vi "rio 9030 jiwon.vi"() -> ()   [LabVIEW 2015]
uses:
  <vilib>/FPGAPlugInAG/cRIO-9030/niLvFpga_Open_cRIO-9030.vi
  <vilib>/rvi/interface/common/dynamic/niFpgaDynamicAddResources.vi
  <vilib>/FPGAPlugInAG/Dynamic/niLvFpga_Abort_Dynamic.vi
  <vilib>/FPGAPlugInAG/Dynamic/niLvFpga_Run_Dynamic.vi
  rio_Global.vi
  <vilib>/Utility/error.llb/Error Cluster From Error Code.vi
  <vilib>/rvi/errors/niLvFpgaAdjustHostInterfaceError.vi
  <vilib>/Analysis/Matrix/Numeric/Conversions/Array To Matrix - RA2.vi
  <vilib>/Analysis/Matrix/Numeric/Multiply/Multiply - RM,RM.vi
  <vilib>/Analysis/Matrix/Numeric/Add/Add - RM,RM.vi
  <vilib>/Analysis/baseanly.llb/Real Inverse Matrix.vi
  <vilib>/Analysis/Matrix/Numeric/Subtract/Subtract - RM,RM.vi
  <vilib>/Analysis/Matrix/Numeric/Conversions/Array To Matrix - RA.vi
  <vilib>/Analysis/Matrix/Numeric/Multiply/Multiply - R,RM.vi
  <vilib>/Analysis/Matrix/Numeric/Conversions/Matrix To Array - RM.vi
  <vilib>/rvi/interface/nirviOpenFPGA/nirviOpenFPGA.xnode
  FPGA Bitfiles/autonomous_FPGATarget4_fpga1_rudp+OsNkSQ.lvbitx
  samsung/fpga 1.vi
  <vilib>/rvi/interface/nirviMethod/nirviMethod.xnode
  <vilib>/rvi/interface/nirviReadWriteControl/nirviReadWriteControl.xnode
  <vilib>/FPGAPlugInAG/Dynamic/niLvFpga_ReadFifo_Dynamic.vi
  <vilib>/rvi/errors/niLvFpgaMergeErrorWithErrorCode.vi
  <vilib>/Analysis/Matrix/NI_Matrix.lvlib
  <vilib>/Analysis/NI_AALBase.lvlib
  <vilib>/rvi/interface/Simulation/niFpgaSimulationCallBeginRW.vi
  NiFpgaLv.dll
  <vilib>/addons/control/pid/NI_PID_pid.lvlib
  <vilib>/ptbypt/NI_PtbyPt.lvlib
  <vilib>/addons/control/pid/pid.llb/PID (DBL).vi
panel:
  in  "s":bool
  in  "Radio Buttons":enum32{"-480", "0", "480"}(radio)
  in  "Ref_str_ang":dbl
  out "error":dbl
  in  "STEERING PID_gain_Avante":dbl[](array[numeric])=[0.02, 6.5, 0.003]
  in  "STEERING PID_gain_Santafe":dbl[](array[numeric])=[0.02, 6.5, 0.003]
  out "map name":T1(ring)=enum."KAIST"
  out "Waveform Chart 3":dbl(graph)
  in  "lpf gain 2":dbl=0.8 format="%#_13g"
  out "con_dt":dbl
  in  "lpf gain":dbl=0.8 format="%#_13g"
  out "Waveform Chart 2":dbl(graph)
  in  "Dial":dbl(knob) min=-360.0 max=360.0 step=5.0 scale=-360.0..360.0
  out "FPGA":refnum<k20>
  out "C_yaw_rate":dbl
  in  "speed control":bool
  out "C_MCP":dbl
  out "C_APV":dbl
  out "Ref_VS":dbl
  out "XY Graph":cluster{"Y":dbl[], "Y":dbl[]}[](graph)=[{"Y"=[1.82421875, 1.8301353427767753, 1.835194070339203, 1.8394013252854347, 1.8427635002136231, 1.84528698772192, 1.8469781804084777, 1.8478434708714486, 1.8478892517089844, 1.8471219155192375, 1.84554785490036, 1.8431734624505043, 1.8400051307678222, 1.8360492524504661, 1.8313122200965881, 1.8258004263043404, 1.819520263671875, 1.8124781247973443, 1.8046804022789003, 1.796133488714695, 1.7868437767028809, 1.77681765884161, 1.7660615277290344, 1.7545817759633064, 1.742384796142578, 1.7294769808650017, 1.7158647227287291, 1.701554414331913, 1.686552448272705, 1.6708652171492577, 1.654499113559723, 1.637460530102253, 1.619755859375, 1.6013914939761162, 1.5823738265037537, 1.5627092495560646, 1.5424041557312012, 1.5214649376273155, 1.4998979878425598, 1.4777096989750862, 1.4549064636230469, 1.431494674384594, 1.4074807238578795, 1.3828710046410562, 1.3576719093322753, 1.3318898305296898, 1.3055311608314515, 1.2786022928357124, 1.251109619140625, 1.2230595323443412], "Y"=[0.0, 0.5, 1.0, 1.5, 2.0, 2.5, 3.0, 3.5, 4.0, 4.5, 5.0, 5.5, 6.0, 6.5, 7.0, 7.5, 8.0, 8.5, 9.0, 9.5, 10.0, 10.5, 11.0, 11.5, 12.0, 12.5, 13.0, 13.5, 14.0, 14.5, 15.0, 15.5, 16.0, 16.5, 17.0, 17.5, 18.0, 18.5, 19.0, 19.5, 20.0, 20.5, 21.0, 21.5, 22.0, 22.5, 23.0, 23.5, 24.0, 24.5]}, {"Y"=[-1.22265625, -1.2167396572232247, -1.211680929660797, -1.2074736747145653, -1.2041114997863769, -1.20158801227808, -1.1998968195915223, -1.1990315291285514, -1.1989857482910156, -1.1997530844807625, -1.20132714509964, -1.2037015375494957, -1.2068698692321778, -1.2108257475495339, -1.2155627799034119, -1.2210745736956596, -1.227354736328125, -1.2343968752026557, -1.2421945977210997, -1.250741511285305, -1.2600312232971191, -1.27005734115839, -1.2808134722709656, -1.2922932240366936, -1.304490203857422, -1.3173980191349983, -1.3310102772712709, -1.345320585668087, -1.360322551727295, -1.3760097828507423, -1.392375886440277, -1.409414469897747, -1.427119140625, -1.4454835060238838, -1.4645011734962463, -1.4841657504439354, -1.5044708442687988, -1.5254100623726845, -1.5469770121574402, -1.5691653010249138, -1.5919685363769531, -1.615380325615406, -1.6393942761421205, -1.6640039953589438, -1.6892030906677247, -1.7149851694703102, -1.7413438391685485, -1.7682727071642876, -1.795765380859375, -1.8238154676556588, -1.8524165749549866, -1.8815623101592065, -1.911246280670166, -1.9414620938897134, -1.972203357219696, -2.003463678061962, -2.0352366638183597, -2.0675159218907355, -2.1002950596809384, -2.1335676845908162, -2.167327404022217, -2.2015678253769875, -2.2362825560569766, -2.2714652034640315, -2.307109375, -2.3432086780667305, -2.3797567200660703, -2.4167471083998677, -2.4541734504699706, -2.4920293536782263, -2.530308425426483, -2.5690042731165885, -2.6081105041503907, -2.647620725929737, -2.687528545856476, -2.7278275713324547, -2.7685114097595216, -2.809573668539524, -2.8510079550743104, -2.892807876765728, -2.934967041015625, -2.977479055225849, -3.020337526798248, -3.0635360631346704, -3.107068271636963, -3.150927759706974, -3.1951081347465515, -3.2396030041575434, -3.284405975341797, -3.3295106557011604, -3.3749106526374817, -3.4205995735526087, -3.466571025848389, -3.51281861692667, -3.5593359541893004], "Y"=[0.0, 0.5, 1.0, 1.5, 2.0, 2.5, 3.0, 3.5, 4.0, 4.5, 5.0, 5.5, 6.0, 6.5, 7.0, 7.5, 8.0, 8.5, 9.0, 9.5, 10.0, 10.5, 11.0, 11.5, 12.0, 12.5, 13.0, 13.5, 14.0, 14.5, 15.0, 15.5, 16.0, 16.5, 17.0, 17.5, 18.0, 18.5, 19.0, 19.5, 20.0, 20.5, 21.0, 21.5, 22.0, 22.5, 23.0, 23.5, 24.0, 24.5, 25.0, 25.5, 26.0, 26.5, 27.0, 27.5, 28.0, 28.5, 29.0, 29.5, 30.0, 30.5, 31.0, 31.5, 32.0, 32.5, 33.0, 33.5, 34.0, 34.5, 35.0, 35.5, 36.0, 36.5, 37.0, 37.5, 38.0, 38.5, 39.0, 39.5, 40.0, 40.5, 41.0, 41.5, 42.0, 42.5, 43.0, 43.5, 44.0, 44.5, 45.0, 45.5, 46.0, 46.5, 47.0]}, {"Y"=[-0.94, 0.94, 0.94, -0.94, -0.94], "Y"=[-3.2, -3.2, 1.5, 1.5, -3.2]}, {"Y"=[1.984375, 1.978057861328125, 1.9718017578125, 1.965606689453125, 1.95947265625], "Y"=[0.0, 0.5, 1.0, 1.5, 2.0]}, {"Y"=[-5.28125, -5.267578125, -5.25390625, -5.240234375, -5.2265625], "Y"=[0.0, 0.5, 1.0, 1.5, 2.0]}]
  out "x_view":dbl[](array[numeric])=[0.0, 0.5, 1.0, 1.5, 2.0, 2.5, 3.0, 3.5, 4.0, 4.5, 5.0, 5.5, 6.0, 6.5, 7.0, 7.5, 8.0, 8.5, 9.0, 9.5, 10.0, 10.5, 11.0, 11.5, 12.0, 12.5, 13.0, 13.5, 14.0, 14.5, 15.0, 15.5, 16.0, 16.5, 17.0, 17.5, 18.0, 18.5, 19.0, 19.5, 20.0, 20.5, 21.0, 21.5, 22.0, 22.5, 23.0, 23.5, 24.0, 24.5, 25.0, 25.5, 26.0, 26.5, 27.0, 27.5, 28.0, 28.5, 29.0, 29.5, 30.0, 30.5, 31.0, 31.5, 32.0, 32.5, 33.0, 33.5, 34.0, 34.5, 35.0, 35.5, 36.0, 36.5, 37.0, 37.5, 38.0, 38.5, 39.0, 39.5, 40.0, 40.5, 41.0, 41.5, 42.0, 42.5, 43.0, 43.5, 44.0, 44.5, 45.0, 45.5, 46.0, 46.5, 47.0, 47.5, 48.0, 48.5, 49.0, 49.5, 50.0, 50.5, 51.0, 51.5, 52.0, 52.5, 53.0, 53.5, 54.0, 54.5, 55.0, 55.5, 56.0, 56.5, 57.0, 57.5, 58.0, 58.5, 59.0, 59.5, 60.0, 60.5, 61.0, 61.5, 62.0, 62.5, 63.0, 63.5, 64.0, 64.5, 65.0, 65.5, 66.0, 66.5, 67.0, 67.5, 68.0, 68.5, 69.0, 69.5, 70.0, 70.5, 71.0, 71.5, 72.0, 72.5, 73.0, 73.5, 74.0, 74.5, 75.0, 75.5, 76.0, 76.5, 77.0, 77.5, 78.0, 78.5, 79.0, 79.5, 80.0, 80.5, 81.0, 81.5, 82.0, 82.5, 83.0, 83.5, 84.0, 84.5, 85.0, 85.5, 86.0, 86.5, 87.0, 87.5, 88.0, 88.5, 89.0, 89.5, 90.0, 90.5, 91.0, 91.5, 92.0, 92.5, 93.0, 93.5, 94.0, 94.5, 95.0, 95.5, 96.0, 96.5, 97.0, 97.5, 98.0, 98.5, 99.0, 99.5, 100.0, 100.5, 101.0, 101.5, 102.0, 102.5, 103.0, 103.5, 104.0, 104.5, 105.0, 105.5, 106.0, 106.5, 107.0, 107.5, 108.0, 108.5, 109.0, 109.5, 110.0, 110.5, 111.0, 111.5, 112.0, 112.5, 113.0, 113.5, 114.0, 114.5, 115.0, 115.5, 116.0, 116.5, 117.0, 117.5, 118.0, 118.5, 119.0, 119.5, 120.0, 120.5, 121.0, 121.5, 122.0, 122.5, 123.0, 123.5, 124.0, 124.5, 125.0, 125.5, 126.0, 126.5, 127.0, 127.5, 128.0]
  in  "Manual Steering torque":dbl(slide) min=-0.9 max=0.9 step=0.01 scale=-0.9..0.9
  out "T init":i32
  out "T out":i32
  out "PWM GAS":dbl=1000.0 min=1000.0 max=2000.0 step=1.0
  out "Mobileye_time 50":u32
  out "H_GPS":dbl
  out "vgain":dbl=1.0
  out "vcount":u64=1
  out "hbias":dbl
  out "hcount":u64=1
  out "get heading":bool
  out "get position":bool
  out "heading error":dbl
  out "h_gps":dbl
  out "rt":dbl
  out "pos error":dbl
  out "POS init":bool
  out "Heading":dbl
  out "pos":dbl[](array[numeric])
  in  "GPS init":bool=TRUE
  out "pos_gps":dbl[](array[numeric]) format="%#_19f"
  out "dt":dbl
  out "Pos_time 10":i32
  out "ecef ref":dbl[](array[numeric])
  in  "Velocity input":bool
  in  "Manual Speed":dbl=1.0
  in  "Steer input":bool=TRUE
  out "Run":bool
  out "Auto":bool
  out "E - STOP":bool
  out "Con_time 10":i32
  out "VS_CAN":dbl
  out "CAN_time 10":u32
  out "gps1":refnum<visa-resource-name>
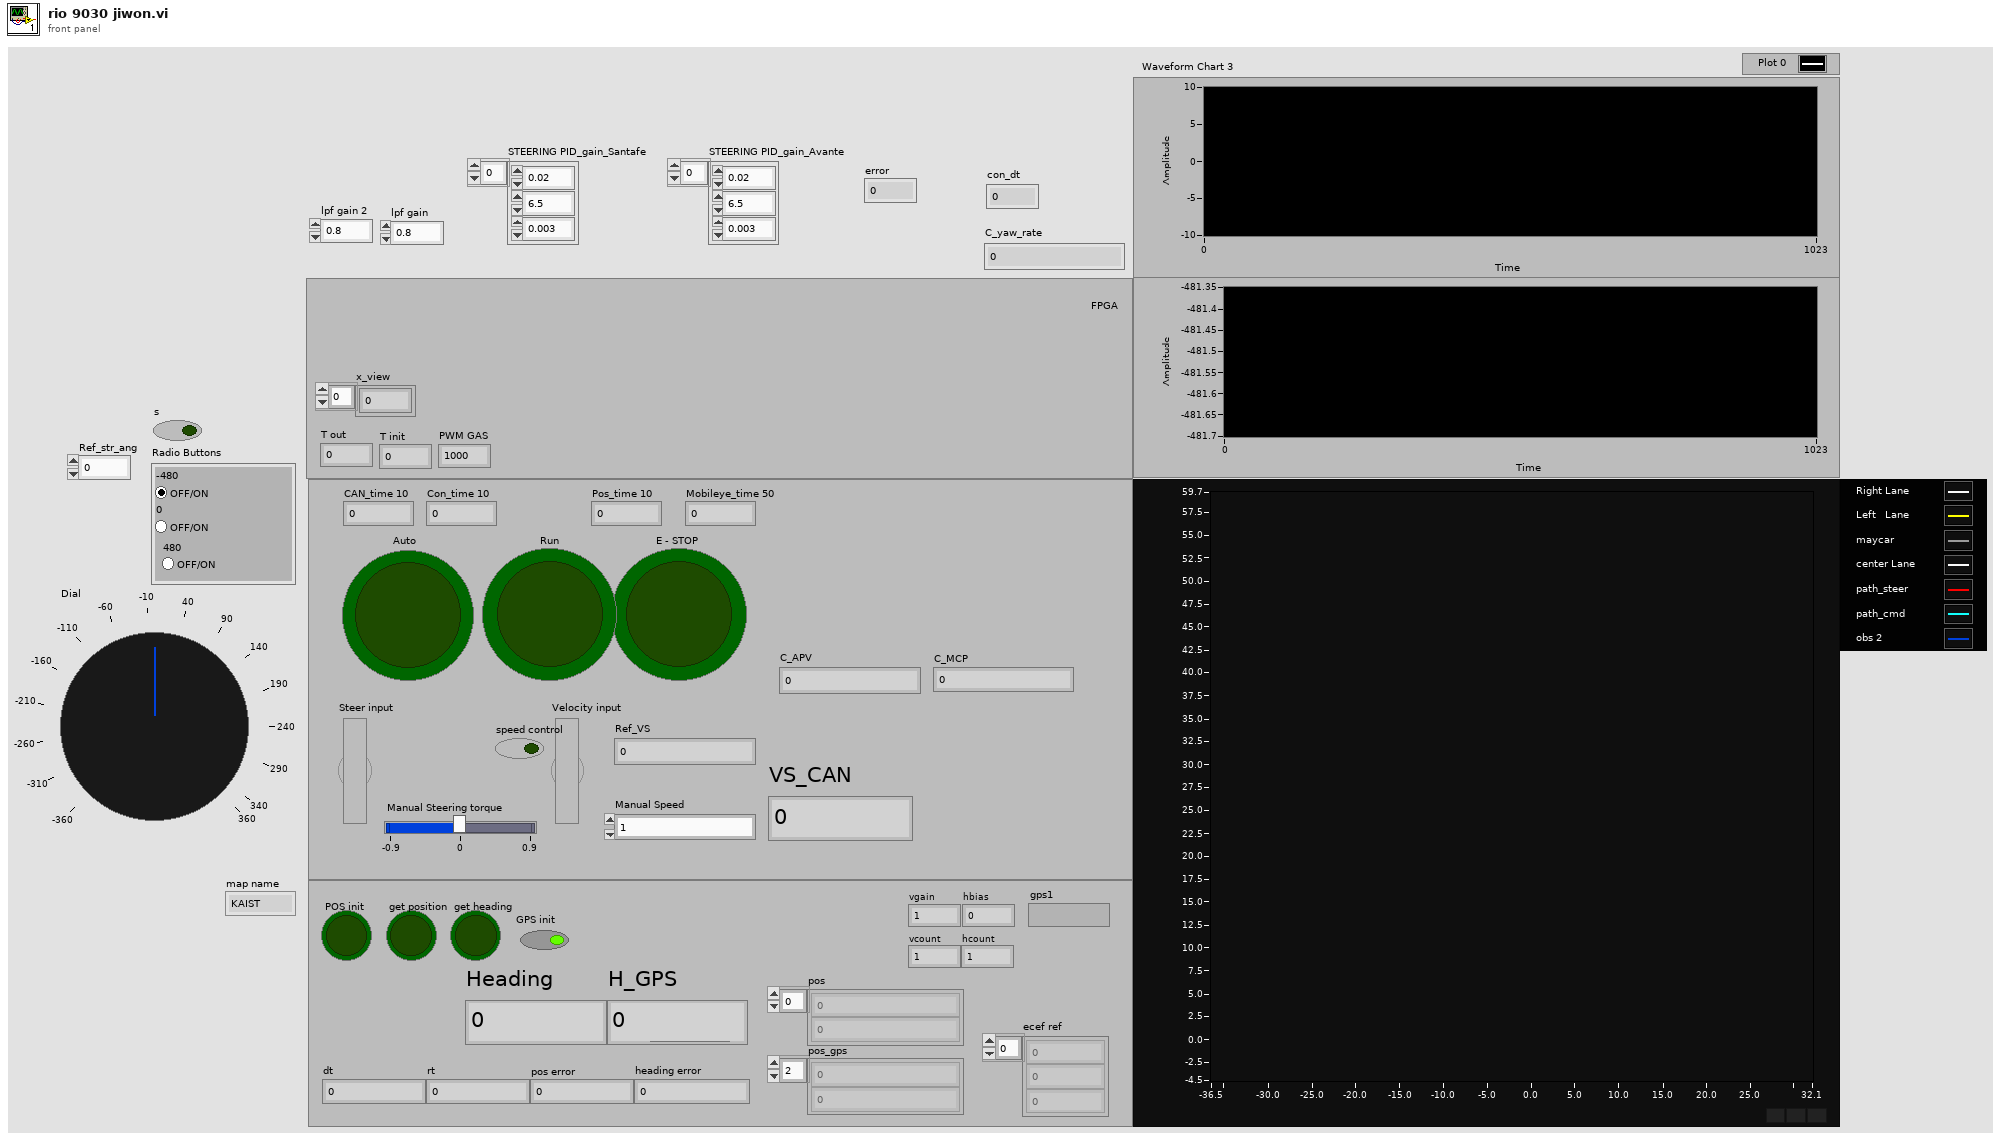
[diagram p1: front panel]
types:
  T1 = enum32{"Namyang", "Hyundai", "KAIST", "Ajou", "Munji", "Airforce", "Car", "KATRI", "Samsung", "Coex", "Gwangnaru", "Inje", "sinjin"}
  T2 = cluster{"proportional gain (Kc)":dbl, "integral time (Ti, min)":dbl, "derivative time (Td, min)":dbl}
  T3 = cluster{"connection ID":refnum<k16>, "net address":u32, "port":u16}
  T4 = cluster{"hash":i64, "sys time":i64, "ref_vel":dbl, "ref_steer":dbl, "alert":u8}
  T5 = cluster{"hash":i64, "sys time":i64, "ref_vel":dbl, "ref_steer":dbl}
  T6 = cluster{"hash":i64, "sys time":i64, "Auto":bool, "Run":bool, "Solenoid":bool, "T lim":bool, "brk_enc":u8, "B PWM":u16, "T PWM":u16, "ref_vel":dbl, "ref_bkr_enc":dbl, "ref_apv":dbl, "ref_steer":dbl, "net address":u32}
  T7 = cluster{"identifier":u32, "timestamp":timestamp, "payload":u8[]}
  T8 = cluster{"timestamp high":u32, "timestamp low":u32, "identifier":u32, "type":enum8{"Data Frame", "Remote Frame", "(reserved)", "(reserved) ", "(reserved)  ", "(reserved)   ", "Bus Error", "Transceiver Fault"}, "info A":u8, "info B":u8, "data length":u8, "data":u8[]}
  T9 = cluster{"hash":i64, "sys time":i64, "size":i32, "data":u8[]}
  T10 = cluster{"hash":i64, "sys time":i64, "time":dbl, "yaw_rate":dbl, "mdps torque":dbl, "mdps str_ang":dbl, "VS_CAN":dbl, "lat_accel":dbl, "mcp":dbl, "accel pedal value":dbl, "tps":dbl, "odometer":dbl, "battery voltage":dbl, "WHL_SPD_RR":dbl, "WHL_SPD_RL":dbl, "WHL_SPD_FR":dbl, "WHL_SPD_FL":dbl}
  T11 = typedef "NI_Matrix.lvlib/RealMatrix.ctl" = dbl[][]
  T12 = cluster{"hash":i64, "sys time":i64, "dt":dbl, "x":dbl, "y":dbl, "speed":dbl, "heading":dbl, "yaw_rate":dbl}
  T13 = cluster{"Real 2D Array[0]":dbl, "Real 2D Array[1]":dbl, "Real 2D Array[2]":dbl, "Real 2D Array[3]":dbl, "Real 2D Array[4]":dbl}
  T14 = cluster{"hash":i64, "sys time":i64, "time":dbl, "x":dbl, "y":dbl, "h":dbl, "numSV":i32, "postype":i32, "lag":i32, "hordev":dbl, "lat":dbl, "lon":dbl, "hgt":dbl, "map_idx":i32}
  T15 = cluster{"output[0]":dbl, "output[1]":dbl, "output[2]":dbl, "output[3]":dbl, "output[4]":dbl, "output[5]":dbl, "output[6]":dbl, "output[7]":dbl, "output[8]":dbl, "output[9]":dbl, "output[10]":dbl, "output[11]":dbl, "output[12]":dbl, "output[13]":dbl, "output[14]":dbl}
  T16 = cluster{"hash":i64, "sys time":i64, "time":dbl, "speed":dbl, "heading":dbl, "lat":dbl, "lon":dbl}
  T17 = cluster{"output[0]":dbl, "output[1]":dbl, "output[2]":dbl, "output[3]":dbl, "output[4]":dbl, "output[5]":dbl, "output[6]":dbl}
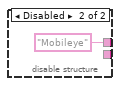
[diagram p2: hidden frame]
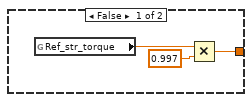
[diagram p3: hidden frame]
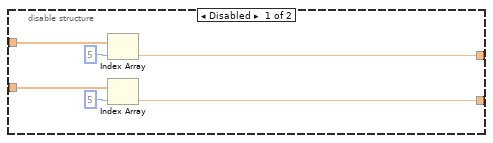
[diagram p4: hidden frame]
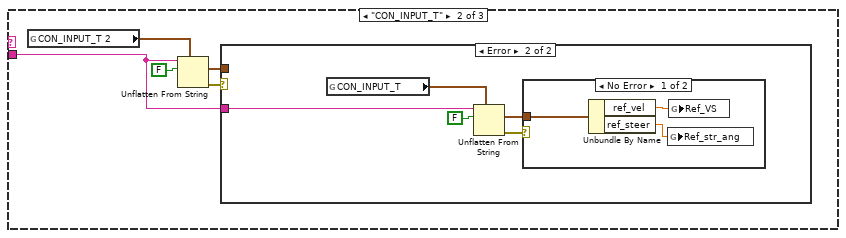
[diagram p6: hidden frame]
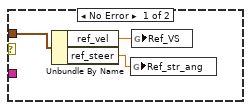
[diagram p7: hidden frame]
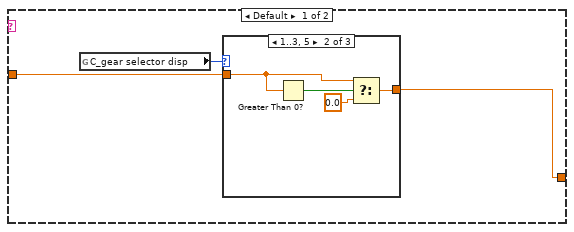
[diagram p10: hidden frame]
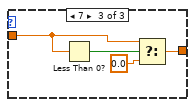
[diagram p12: hidden frame]
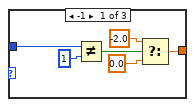
[diagram p13: hidden frame]
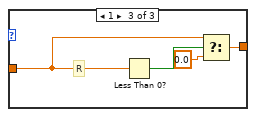
[diagram p16: hidden frame]
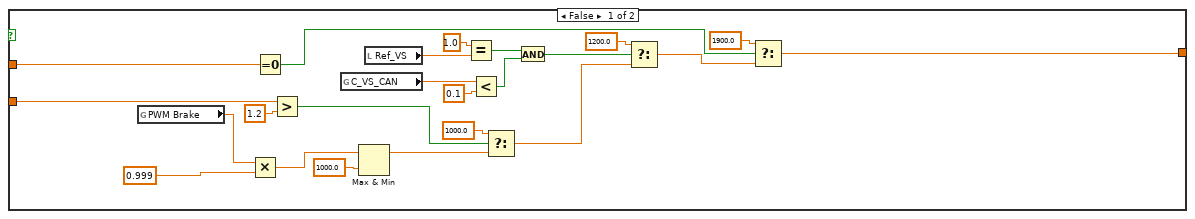
[diagram p17: hidden frame]
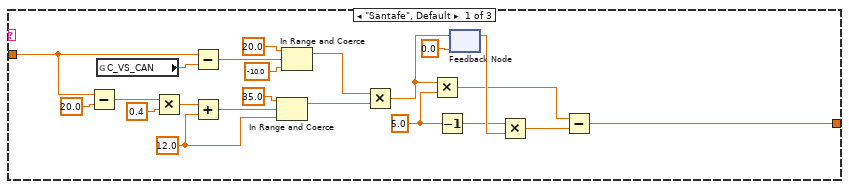
[diagram p19: hidden frame]
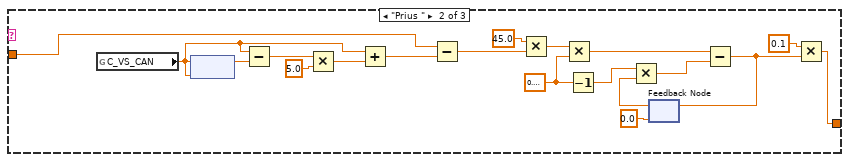
[diagram p20: hidden frame]
diagram:
  n1 = flat-sequence {
    frame #0 {
      n2 = local write "Manual Steering torque"(0.0 ("Ref_vel_planner")) -> ()
      n3 = local write "Velocity input"(FALSE ("GPS init")) -> ()
      n4 = local write "Steer input"(FALSE ("Steer input")) -> ()
      n5 = local write "Manual Speed"(20.0 ("manual Speed")) -> ()
      n6 = global write "rio_Global.vi" "lane width"(3.5 ("lane width")) -> ()
    }
    frame #1 {
      n7 = while {
        stop <- FALSE stop-if-true
        n8 = flat-sequence {
          tunnel: [w127] -> w7
          tunnel: w7 -> [w180]
          frame #0 {
            n9 = Wait Until Next ms Multiple(millisecond multiple=u32 10) -> (millisecond timer value=w12:u32)
            n10 = feedback #1(w12) -> (w11:u32)
            n11 = feedback-in #1(w12) -> ()
            n12 = Subtract(x=w12, y=w11) -> (x-y=w10:u32)
            n13 = To Long Integer(number=w10) -> (32bit integer=→"Con_time 10":i32)
          }
          frame #1 {
            n14 = disable-structure shown="Enabled" {
              disable-tunnel: [w17 "Mobileye" ("ID")] -> w15
              disable-tunnel: [w16 _] -> w14
              frame Enabled {
                n15 = global read "rio_Global.vi" "LCM PC"() -> (w18:T3)
                n16 = call "LCM_read.vi"("LCM"=w18) -> ("data"=w16:string, "ID"=w17:string)  [unwired: 7 in, 2 out]
              }
              frame Disabled {
              }
            }
            n17 = case shown="\"Mobileye\"" w15 {
              tunnel: w14 -> [_ w111 _]
              frame "Mobileye" {
                n18 = flat-sequence {
                  frame #0 {
                    w26 = 2 ("index")
                    w29 = 2 ("index")
                    n19 = global read "rio_Global.vi" "M_lane_right"() -> (w21:dbl[])
                    n20 = global read "rio_Global.vi" "M_lane_left"() -> (w22:dbl[])
                    n21 = Index Array(array=w22, index=w29) -> (element=w28:dbl)
                    n22 = Index Array(array=w21, index=w26) -> (element=w27:dbl)
                    n23 = Greater Or Equal?(x=w28, y=w29) -> (x >= y?=w23:bool)
                    n24 = Greater Or Equal?(x=w27, y=w26) -> (x >= y?=w24:bool)
                    n25 = Or(x=w23, y=w24) -> (x .or. y?=w25:bool)
                    n26 = case shown="True" w25 {
                      tunnel: w24 -> [_ w57]
                      tunnel: [w30 w46] -> w20
                      tunnel: w23 -> [_ w60]
                      tunnel: w22 -> [_ w51]
                      tunnel: w21 -> [_ w50]
                      frame False {
                        n27 = global read "rio_Global.vi" "Ref_str_torque"() -> (w31:dbl)
                        n28 = Multiply(x=w31, y=0.997) -> (x*y=w30:dbl)
                      }
                      frame True {
                        n29 = disable-structure shown="Enabled" {
                          disable-tunnel: [w65 w68] -> w56
                          disable-tunnel: [w64 w90] -> w54
                          disable-tunnel: w51 -> [w63 w99]
                          disable-tunnel: w50 -> [w62 w69]
                          frame Disabled {
                            n30 = Index Array(array=w63, index=5) -> (element=w64:dbl)
                            n31 = Index Array(array=w62, index=5) -> (element=w65:dbl)
                          }
                          frame Enabled {
                            n32 = global read "rio_Global.vi" "C_VS_CAN"() -> (w98:dbl)
                            n33 = global read "rio_Global.vi" "C_VS_CAN"() -> (w74:dbl)
                            n34 = In Range and Coerce(upper limit=45.0, x=w98, lower limit=15.0) -> (coerced(x)=w87:dbl)  [unwired: 1 out]
                            n35 = In Range and Coerce(upper limit=45.0, x=w74, lower limit=15.0) -> (coerced(x)=w84:dbl)  [unwired: 1 out]
                            n36 = Index Array(array=w99, index #1=7 ("index"), index #2=6 ("index"), index #3=9 ("index"), index #4=5 ("index")) -> (element #1=w95:dbl, element #2=w88:dbl, element #3=w86:dbl, element #4=w91:dbl)
                            n37 = Index Array(array=w69, index #1=7 ("index"), index #2=6 ("index"), index #3=9 ("index"), index #4=5 ("index")) -> (element #1=w77:dbl, element #2=w83:dbl, element #3=w85:dbl, element #4=w81:dbl)
                            n38 = Square(x=w87) -> (x^2=w89:dbl)
                            n39 = Square(x=w84) -> (x^2=w82:dbl)
                            n40 = Multiply(x=w89, y=w88) -> (x*y=w93:dbl)
                            n41 = Multiply(x=w87, y=w86) -> (x*y=w92:dbl)
                            n42 = Multiply(x=w82, y=w83) -> (x*y=w79:dbl)
                            n43 = Multiply(x=w84, y=w85) -> (x*y=w80:dbl)
                            n44 = Compound Arithmetic op=MULTIPLY(w95, w89, w87) -> (w94:dbl)
                            n45 = Compound Arithmetic op=MULTIPLY(w77, w82, w84) -> (w78:dbl)
                            n46 = Compound Arithmetic op=ADD(w94, w93, w92, w91) -> (w90:dbl)
                            n47 = Compound Arithmetic op=ADD(w78, w79, w80, w81) -> (w68:dbl)
                          }
                        }
                        n48 = global read "rio_Global.vi" "C_VS_CAN"() -> (w49:dbl)
                        n49 = global read "rio_Global.vi" "lane width"() -> (w53:dbl)
                        n50 = Square(x=w49) -> (x^2=w48:dbl)
                        n51 = Add(x=w54, y=w53) -> (x+y=w52:dbl)
                        n52 = Subtract(x=w56, y=w53) -> (x-y=w58:dbl)
                        n53 = Divide(x=w48, y=-28800.0) -> (x/y=w45:dbl)
                        n54 = Select(t=w54, s=w60, f=w58) -> (s? t:f=w59:dbl)
                        n55 = Select(t=w56, s=w57, f=w52) -> (s? t:f=w55:dbl)
                        n56 = global read "rio_Global.vi" "C_Right light"() -> (w37:bool)
                        n57 = global read "rio_Global.vi" "C_Left light"() -> (w35:bool)
                        n58 = Negate(x=w59) -> (-x=w61:dbl)
                        n59 = Multiply(x=w45, y=4.499999999999998 ("invgain>1")) -> (x*y=w44:dbl)
                        n60 = Subtract(x=w61, y=w55) -> (x-y=w34:dbl)
                        n61 = Exclusive Or(1:w37, 2:w35) -> (0:w36:bool)
                        n62 = Exponential(1:w44) -> (0:w41:dbl)
                        n63 = case shown="True" w36 {
                          tunnel: w35 -> [_ w110]
                          tunnel: [w104 w105] -> w33
                          tunnel: w34 -> [w104 w107]
                          frame False {
                          }
                          frame True {
                            n64 = Select(t=1.0, s=w110, f=-1.0) -> (s? t:f=w106:dbl)
                            n65 = Add(x=w107, y=w106) -> (x+y=w105:dbl)
                          }
                        }
                        n66 = Multiply(x=w41, y=0.125) -> (x*y=w40:dbl)
                        n67 = Max & Min(x=w40, y=0.01) -> (max(x,y)=w39:dbl)  [unwired: 1 out]
                        n68 = Multiply(x=w33, y=w39) -> (x*y=w46:dbl)
                      }
                    }
                    n69 = global write "rio_Global.vi" "Ref_str_torque"(w20) -> ()
                  }
                }
              }
              frame "CON_INPUT_T" {
                n70 = global read "rio_Global.vi" "CON_INPUT_T 2"() -> (w113:T4)
                n71 = Unflatten From String(type=w113, binary string=w111, data includes array or string size? (T)=FALSE) -> (value=w112:T4, error out=w114:errorcluster)  [unwired: 2 in, 1 out]
                n72 = case shown="Error" w114 {
                  tunnel: w112 -> [w118 _]
                  tunnel: w111 -> [_ w119]
                  frame No Error {
                    n73 = Unbundle By Name(w118) -> ("ref_vel"=w117:dbl, "ref_steer"=w116:dbl)
                    n74 = global write "rio_Global.vi" "Ref_str_ang"(w116) -> ()
                    n75 = global write "rio_Global.vi" "Ref_VS"(w117) -> ()
                  }
                  frame Error {
                    n76 = global read "rio_Global.vi" "CON_INPUT_T"() -> (w121:T5)
                    n77 = Unflatten From String(type=w121, binary string=w119, data includes array or string size? (T)=FALSE) -> (value=w120:T5, error out=w122:errorcluster)  [unwired: 2 in, 1 out]
                    n78 = case shown="No Error" w122 {
                      tunnel: w120 -> [w126 _]
                      frame No Error {
                        n79 = Unbundle By Name(w126) -> ("ref_vel"=w125:dbl, "ref_steer"=w124:dbl)
                        n80 = global write "rio_Global.vi" "Ref_str_ang"(w124) -> ()
                        n81 = global write "rio_Global.vi" "Ref_VS"(w125) -> ()
                      }
                      frame Error {
                      }
                    }
                  }
                }
              }
              frame Default {
              }
            }
          }
          frame #2 {
            n82 = global read "rio_Global.vi" "C_VS_CAN"() -> (→"VS_CAN":dbl)
            n83 = global read "rio_Global.vi" "C_MCP"() -> (→"C_MCP":dbl)
            n84 = global read "rio_Global.vi" "Ref_VS"() -> (w128:dbl)
            n85 = global read "rio_Global.vi" "C_APV"() -> (→"C_APV":dbl)
            n86 = local read "Con_time 10"() -> (w134:i32)
            n87 = global read "rio_Global.vi" "Car_name"() -> (w129:string)
            n88 = Select(t=w128, s="Velocity input", f="Manual Speed") -> (s? t:f=w139:dbl)
            n89 = To Double Precision Float(number=w134) -> (double precision float=w135:dbl)
            n90 = case shown="\"Prius\"" w129 {
              tunnel: w139 -> [w143 w157]
              tunnel: [w142 w158] -> w127
              frame Default {
                n91 = global read "rio_Global.vi" "C_gear selector disp"() -> (w144:u8)
                n92 = case shown="1..3, 5" w144 {
                  tunnel: w143 -> [_ w147 w151]
                  tunnel: [_ w146 w150] -> w142
                  frame 0, Default {
                  }
                  frame 1..3, 5 {
                    n93 = Greater Than 0?(x=w147) -> (x > 0?=w148:bool)
                    n94 = Select(t=w147, s=w148, f=0.0) -> (s? t:f=w146:dbl)
                  }
                  frame 7 {
                    n95 = Less Than 0?(x=w151) -> (x < 0?=w152:bool)
                    n96 = Select(t=w151, s=w152, f=0.0) -> (s? t:f=w150:dbl)
                  }
                }
              }
              frame "Prius" {
                n97 = Sign(1:w157) -> (0:w156:dbl)
                n98 = global read "rio_Global.vi" "C_gear selector disp"() -> (w154:u8)
                n99 = To Long Integer(number=w156) -> (32bit integer=w155:i32)
                n100 = case shown="1" w155 {
                  tunnel: [w160 _ w166] -> w153
                  tunnel: w154 -> [w163 _ w169]
                  frame -1 {
                    n101 = Not Equal?(x=w163, y=u8 1) -> (x != y?=w162:bool)
                    n102 = Select(t=-2.0 ("element"), s=w162, f=0.0) -> (s? t:f=w160:dbl)
                  }
                  frame 0, Default {
                  }
                  frame 1 {
                    n103 = Not Equal?(x=w169, y=u8 3) -> (x != y?=w167:bool)
                    n104 = Select(t=2.0 ("element"), s=w167, f=0.0) -> (s? t:f=w166:dbl)
                  }
                }
                n105 = case shown="3" w154 {
                  tunnel: [_ w171 w176] -> w158
                  tunnel: w157 -> [_ w173 w177]
                  frame 0, Default {
                    # "P,N"
                  }
                  frame 3 {
                    # "D"
                    n106 = Greater Than 0?(x=w173) -> (x > 0?=w174:bool)
                    n107 = Select(t=w173, s=w174, f=0.0) -> (s? t:f=w171:dbl)
                  }
                  frame 1 {
                    # "R"
                    n108 = Less Than 0?(x=w177) -> (x < 0?=w178:bool)
                    n109 = Select(t=w177, s=w178, f=0.0) -> (s? t:f=w176:dbl)
                  }
                }
                n110 = global write "rio_Global.vi" "Shift control"(w153) -> ()
              }
            }
            "Ref_VS" <- w127
            n111 = Multiply(x=w135, y=0.001) -> (x*y=w133:dbl)
            n112 = Max & Min(x=w133, y=0.005) -> (max(x,y)=→"con_dt":dbl)  [unwired: 1 out]
          }
          frame #3 {
            n113 = flat-sequence {
              tunnel: [w192] -> w179
              tunnel: w180 -> [w193]
              frame #0 {
                n114 = global read "rio_Global.vi" "C_VS_CAN"() -> (w195:dbl)
                n115 = Subtract(x=w193, y=w195) -> (x-y=w194:dbl)
                n116 = Less?(x=w194, y=0.0 ("lower limit")) -> (x < y?=w196:bool)
                n117 = case shown="True" w196 {
                  tunnel: [w200 w225] -> w192
                  tunnel: w193 -> [w213 w236]
                  tunnel: w194 -> [w210 w228]
                  frame False {
                    n118 = global read "rio_Global.vi" "PWM Brake"() -> (w220:dbl)
                    n119 = Multiply(x=w220, y=0.999 ("brake relase gain")) -> (x*y=w219:dbl)
                    n120 = Equal To 0?(x=w213) -> (x = 0?=w212:bool)
                    n121 = Greater?(x=w210, y=1.2) -> (0:w217:bool)
                    n122 = global read "rio_Global.vi" "C_VS_CAN"() -> (w203:dbl)
                    n123 = Max & Min(x=w219, y=1000.0) -> (max(x,y)=w215:dbl)  [unwired: 1 out]
                    n124 = local read "Ref_VS"() -> (w208:dbl)
                    n125 = Equal?(x=1.0, y=w208) -> (x = y?=w206:bool)
                    n126 = Less?(x=w203, y=0.1 ("x")) -> (x < y?=w201:bool)
                    n127 = Select(t=1000.0, s=w217, f=w215) -> (s? t:f=w199:dbl)
                    n128 = And(x=w206, y=w201) -> (x .and. y?=w205:bool)
                    n129 = Select(t=1200.0, s=w205, f=w199) -> (s? t:f=w198:dbl)
                    n130 = Select(t=1900.0, s=w212, f=w198) -> (s? t:f=w200:dbl)
                  }
                  frame True {
                    w234 = 0.5 ("gain brake")
                    n131 = Absolute Value(x=w228) -> (abs(x)=w227:dbl)
                    n132 = Threshold 1D Array(2:w227, 3:dbl[] [0.1, 0.5, 1.0, 1.5, 2.0, 3.0, 4.0, 5.0, 6.0, 7.0, 8.0, 9.0, 10.0, 6.5, 7.0, 7.5, 8.0, 8.5, 9.0, 9.5, 10.0]) -> (0:w239:dbl)  [unwired: 1 in]
                    n133 = global read "rio_Global.vi" "PWM Brake"() -> (w232:dbl)
                    n134 = Interpolate 1D Array(1:w239, 2:dbl[] [1250.0, 1270.0, 1290.0, 1300.0, 1350.0, 1400.0, 1450.0, 1500.0, 1550.0, 1700.0, 1750.0, 1900.0, 1900.0]) -> (0:w235:dbl)
                    n135 = Decrement(x=w234) -> (x-1=w233:dbl)
                    n136 = Multiply(x=w235, y=w234) -> (x*y=w230:dbl)
                    n137 = Multiply(x=w233, y=w232) -> (x*y=w231:dbl)
                    n138 = Subtract(x=w230, y=w231) -> (x-y=w226:dbl)
                    n139 = disable-structure shown="Enabled" {
                      disable-tunnel: [w241 w242] -> w223
                      disable-tunnel: w226 -> [w241 w255]
                      disable-tunnel: w227 -> [_ w247]
                      frame Disabled {
                      }
                      frame Enabled {
                        n140 = Multiply(x=w247, y=120.0 ("brake p gain")) -> (x*y=w253:dbl)
                        n141 = local read "con_dt"() -> (w250:dbl)
                        n142 = Add(x=w255, y=w253) -> (x+y=w244:dbl)
                        n143 = Multiply(x=w250, y=4.0) -> (x*y=w249:dbl)
                        n144 = call <vilib>:"Derivative x(t) PtByPt.vi"("initialize"=FALSE, "dt"=w249, "initial condition"=0.0, "x"=w247) -> ("dx/dt"=w245:dbl)  [unwired: 1 out]
                        n145 = Multiply(x=30.0 ("bake d gain"), y=w245) -> (x*y=w243:dbl)
                        n146 = Add(x=w244, y=w243) -> (x+y=w242:dbl)
                      }
                    }
                    n147 = Equal To 0?(x=w236) -> (x = 0?=w237:bool)
                    n148 = In Range and Coerce(upper limit=1900.0, x=w223, lower limit=1000.0) -> (coerced(x)=w221:dbl)  [unwired: 1 out]
                    n149 = Select(t=1900.0, s=w237, f=w221) -> (s? t:f=w225:dbl)
                  }
                }
              }
            }
            n150 = global read "rio_Global.vi" "Car_name"() -> (w181:string)
            n151 = case shown="\"Avante\"" w181 {
              tunnel: [w277 w296 w322] -> w186
              tunnel: w180 -> [w276 w295 w321]
              frame "Santafe", Default {
                w260 = 5.0 ("gain accel")
                w268 = 12.0 ("y")
                n152 = Subtract(x=w276, y=20.0) -> (x-y=w272:dbl)
                n153 = global read "rio_Global.vi" "C_VS_CAN"() -> (w257:dbl)
                n154 = Multiply(x=w272, y=0.4) -> (x*y=w270:dbl)
                n155 = Subtract(x=w276, y=w257) -> (x-y=w256:dbl)
                n156 = Add(x=w270, y=w268) -> (x+y=w269:dbl)
                n157 = In Range and Coerce(upper limit=35.0, x=w269, lower limit=w268) -> (coerced(x)=w266:dbl)  [unwired: 1 out]
                n158 = In Range and Coerce(upper limit=20.0, x=w256, lower limit=-10.0) -> (coerced(x)=w265:dbl)  [unwired: 1 out]
                n159 = Multiply(x=w265, y=w266) -> (x*y=w258:dbl)
                n160 = Multiply(x=w258, y=w260) -> (x*y=w262:dbl)
                n161 = Decrement(x=w260) -> (x-1=w259:dbl)
                n162 = feedback #2(0.0) -> (w263:dbl)
                n163 = feedback-in #2(w258) -> ()
                n164 = Multiply(x=w259, y=w263) -> (x*y=w261:dbl)
                n165 = Subtract(x=w262, y=w261) -> (x-y=w277:dbl)
              }
              frame "Prius " {
                w287 = 0.09999999999999998 ("lpf gain speed")
                n166 = global read "rio_Global.vi" "C_VS_CAN"() -> (w280:dbl)
                n167 = feedback #3(w280) -> (w281:dbl)
                n168 = feedback-in #3(w280) -> ()
                n169 = Subtract(x=w280, y=w281) -> (x-y=w291:dbl)
                n170 = Multiply(x=w291, y=5.0) -> (x*y=w290:dbl)
                n171 = Add(x=w280, y=w290) -> (x+y=w289:dbl)
                n172 = Subtract(x=w295, y=w289) -> (x-y=w294:dbl)
                n173 = Multiply(x=45.0 ("x 2"), y=w294) -> (x*y=w288:dbl)
                n174 = Multiply(x=w288, y=w287) -> (x*y=w285:dbl)
                n175 = Decrement(x=w287) -> (x-1=w286:dbl)
                n176 = feedback #4(0.0) -> (w283:dbl)
                n177 = Multiply(x=w286, y=w283) -> (x*y=w284:dbl)
                n178 = Subtract(x=w285, y=w284) -> (x-y=w279:dbl)
                n179 = feedback-in #4(w279) -> ()
                n180 = Multiply(x=0.1, y=w279) -> (x*y=w296:dbl)
              }
              frame "Avante" {
                n181 = global read "rio_Global.vi" "C_VS_CAN"() -> (w320:dbl)
                n182 = Subtract(x=w321, y=w320) -> (x-y=w319:dbl)
                n183 = In Range and Coerce(upper limit=20.0, x=w319, lower limit=-999.0) -> (coerced(x)=w298:dbl)  [unwired: 1 out]
                n184 = feedback #5(w298) -> (w300:dbl)
                n185 = feedback-in #5(w298) -> ()
                n186 = Absolute Value(x=w298) -> (abs(x)=w306:dbl)
                n187 = feedback #6(0.0) -> (w315:dbl)
                n188 = Multiply(x=w315, y=0.95) -> (x*y=w309:dbl)
                n189 = Multiply(x=w298, y=0.01) -> (x*y=w316:dbl)
                n190 = Subtract(x=w298, y=w300) -> (x-y=w299:dbl)
                n191 = Greater?(x=w306, y=1.0) -> (0:w303:bool)
                n192 = Add(x=w309, y=w316) -> (x+y=w310:dbl)
                n193 = feedback-in #6(w310) -> ()
                n194 = Select(t=w298, s=w303, f=0.0) -> (s? t:f=w313:dbl)
                n195 = Divide(x=w299, y=0.01) -> (x/y=w297:dbl)
                n196 = Build Array(w313, w310, w297) -> (w312:dbl[])
                n197 = Multiply(x=dbl[] [1.0, 25.0, 5.0] ("V_PID_gain_avnate"), y=w312) -> (x*y=w311:dbl[])
                n198 = Add Array Elements(numeric array=w311) -> (sum=w322:dbl)
              }
            }
            n199 = Not Equal To 0?(x=w180) -> (x != 0?=w182:bool)
            n200 = global read "rio_Global.vi" "C_Brake"() -> (w184:bool)
            n201 = local read "T out"() -> (w188:i32)
            n202 = local read "T init"() -> (w189:i32)
            n203 = Greater Or Equal?(x=w189, y=w188) -> (x >= y?=w185:bool)
            n204 = Not(x=w184) -> (.not. x?=w183:bool)
            n205 = Compound Arithmetic op=AND(w185, w183, w182) -> (w187:bool)
            n206 = case shown="True" w187 {
              tunnel: [1000.0 ("Numeric") w338] -> w190
              tunnel: w186 -> [_ w340]
              tunnel: w188 -> [w324 _]
              tunnel: [_ TRUE] -> w191
              frame False {
                n207 = local read "T init"() -> (w325:i32)
                n208 = Less Or Equal?(x=w325, y=w324) -> (x <= y?=w326:bool)
                n209 = case shown="False" w326 {
                  tunnel: w324 -> [_ w329]
                  frame False {
                    n210 = local write "T init"(1 ("T init")) -> ()
                  }
                  frame True {
                    n211 = local read "T init"() -> (w332:i32)
                    n212 = Increment(x=w332) -> (x+1=w331:i32)
                    n213 = Max & Min(x=w331, y=w329) -> (min(x,y)=w330:i32)  [unwired: 1 out]
                    n214 = local write "T init"(w330) -> ()
                  }
                }
              }
              frame True {
                n215 = To Long Integer(number=w340) -> (32bit integer=w342:i32)
                n216 = Multiply(x=10.0, y=w340) -> (x*y=w337:dbl)
                n217 = Add(x=w342, y=20) -> (x+y=w344:i32)
                "T out" <- w344
                n218 = Add(x=w337, y=1000.0 ("PWM GAS")) -> (x+y=w335:dbl)
                n219 = Increment(x=w344) -> (x+1=→"T init":i32)
                n220 = In Range and Coerce(upper limit=1600.0, x=w335, lower limit=1000.0 ("x")) -> (coerced(x)=w338:dbl)  [unwired: 1 out]
              }
            }
            "PWM GAS" <- w190
            n221 = global write "rio_Global.vi" "Solenoid"(w191) -> ()
            n222 = global write "rio_Global.vi" "PWM GAS"(w190) -> ()
            n223 = disable-structure shown="Enabled" {
              disable-tunnel: w179 -> [w323 _]
              frame Enabled {
                n224 = global write "rio_Global.vi" "PWM Brake"(w323) -> ()
              }
              frame Disabled {
              }
            }
          }
          frame #4 {
            n225 = disable-structure shown="Disabled" {
              disable-tunnel: [w459 "Dial" "Ref_str_ang"] -> w347
              frame Enabled {
                n226 = To Double Precision Float(number="Radio Buttons") -> (double precision float=w456:dbl)
                n227 = Decrement(x=w456) -> (x-1=w455:dbl)
                n228 = global read "rio_Global.vi" "Ref_str_ang"() -> (w462:dbl)
                n229 = Multiply(x=w455, y=480.0) -> (x*y=w457:dbl)
                n230 = Select(t=w462, s="s", f=w457) -> (s? t:f=w459:dbl)
              }
              frame Disabled {
              }
              frame Disabled {
              }
            }
            n231 = disable-structure shown="Enabled" {
              disable-tunnel: [_ w406] -> w346
              disable-tunnel: w347 -> [_ w391]
              frame Disabled {
                w376 = 0.6000000000000001 ("y")
                n232 = Absolute Value() -> (x=w351:dbl, abs(x)=w370:dbl)
                n233 = Not A Number/Path/Refnum?(number/path/refnum=w351) -> (NaN/Path/Refnum?=w379:bool)
                n234 = Select(t=0.0, s=w379, f=w351) -> (s? t:f=w378:dbl)
                n235 = Multiply(x=w370, y=-0.02) -> (x*y=w368:dbl)
                n236 = Add(x=w368, y=1.1) -> (x+y=w366:dbl)
                n237 = In Range and Coerce(upper limit=0.22, x=w366, lower limit=0.08) -> (coerced(x)=w363:dbl)  [unwired: 1 out]
                n238 = global read "rio_Global.vi" "C_mdps str_ang"() -> (w355:dbl)
                n239 = Negate(x=w363) -> (-x=w361:dbl)
                n240 = Bundle By Name(cluster=T2 {"proportional gain (Kc)"=-0.1, "integral time (Ti, min)"=0.0, "derivative time (Td, min)"=0.0} ("PID gains"), "proportional gain (Kc)"=w361) -> (w360:T2)
                n241 = Not A Number/Path/Refnum?(number/path/refnum=w355) -> (NaN/Path/Refnum?=w383:bool)
                n242 = Select(t=0.0, s=w383, f=w355) -> (s? t:f=w381:dbl)
                n243 = call-poly <vilib>:"PID.vi"("output range"=cluster{"output high":dbl, "output low":dbl} {"output high"=5.0, "output low"=-5.0}, "dt (s)"=-1.0, "PID gains"=w360, "process variable"=w381, "setpoint"=w378) -> ("output"=w377:dbl)  [unwired: 5 in, 1 out]
                n244 = Decrement(x=w376) -> (x-1=w375:dbl)
                n245 = Multiply(x=w377, y=w376) -> (x*y=w372:dbl)
                n246 = global read "rio_Global.vi" "C_mdps torque"() -> (w353:dbl)
                n247 = feedback #7(0.0) -> (w374:dbl)
                n248 = Multiply(x=w375, y=w374) -> (x*y=w373:dbl)
                n249 = Subtract(x=w372, y=w373) -> (x-y=w357:dbl)
                n250 = Not A Number/Path/Refnum?(number/path/refnum=w357) -> (NaN/Path/Refnum?=w359:bool)
                n251 = Select(t=0.0, s=w359, f=w357) -> (s? t:f=w356:dbl)
                n252 = feedback-in #7(w356) -> ()
                n253 = Multiply(x=-0.05 ("x 5"), y=w353) -> (x*y=w352:dbl)
                n254 = Multiply(x=0.1 ("x 2"), y=w356) -> (x*y=w384:dbl)
                n255 = Add(x=w384, y=w352) -> ()  [unwired: 1 out]
              }
              frame Enabled {
                n256 = global read "rio_Global.vi" "C_mdps str_ang"() -> (w401:dbl)
                n257 = disable-structure shown="Enabled" {
                  disable-tunnel: [w425 w434] -> w390
                  disable-tunnel: w401 -> [w424 w434]
                  frame Enabled {
                    n258 = flat-sequence {
                      tunnel: w424 -> [w433]
                      tunnel: [w427] -> w425
                      frame #0 {
                        n259 = Multiply(x=w433, y="lpf gain 2") -> (x*y=w431:dbl)
                        n260 = Decrement(x="lpf gain 2") -> (x-1=w432:dbl)
                        n261 = feedback #8(0.0) -> (w429:dbl)
                        n262 = Multiply(x=w432, y=w429) -> (x*y=w430:dbl)
                        n263 = Subtract(x=w431, y=w430) -> (x-y=w427:dbl)
                        n264 = feedback-in #8(w427) -> ()
                      }
                    }
                  }
                  frame Disabled {
                  }
                }
                n265 = local read "con_dt"() -> (w404:dbl)
                n266 = Multiply(x=w404, y=4.0) -> (x*y=w403:dbl)
                n267 = Add(x=w391, y=w390) -> (x+y=w405:dbl)
                "error" <- w405
                n268 = call <vilib>:"Derivative x(t) PtByPt.vi"("initialize"=FALSE, "dt"=w403, "initial condition"=0.0, "x"=w390) -> ("dx/dt"=w392:dbl)  [unwired: 1 out]
                n269 = flat-sequence {
                  tunnel: w405 -> [w436]
                  tunnel: [w435] -> w394
                  frame #0 {
                    n270 = disable-structure shown="Enabled" {
                      disable-tunnel: w436 -> [w438 w443]
                      disable-tunnel: [w437 w443] -> w435
                      frame Enabled {
                        n271 = Absolute Value(x=w438) -> (abs(x)=w442:dbl)
                        n272 = Greater?(x=w442, y=0.4) -> (0:w440:bool)
                        n273 = Select(t=w438, s=w440, f=0.0) -> (s? t:f=w437:dbl)
                      }
                      frame Disabled {
                      }
                    }
                    "Waveform Chart 2" <- w435
                  }
                }
                n274 = global read "rio_Global.vi" "Car_name"() -> (w389:string)
                n275 = local read "con_dt"() -> (w411:dbl)
                n276 = case shown="\"Avante\"" w389 {
                  tunnel: ["STEERING PID_gain_Avante" "STEERING PID_gain_Santafe"] -> w388
                  frame "Avante" {
                  }
                  frame "Santafe", Default {
                  }
                }
                n277 = feedback #9(0.0) -> (w410:dbl)
                n278 = Add(x=w394, y=w410) -> (x+y=w412:dbl)
                n279 = call <vilib>:"Integral x(t) PtByPt.vi"("initialize"=FALSE, "dt"=w411, "initial condition"=0.0, "x"=w412) -> ("integral x(t)"=w419:dbl)  [unwired: 1 out]
                n280 = Compound Arithmetic op=MULTIPLY(w419, 0.01 ("x")) -> (w400:dbl)
                n281 = Build Array(w394, w400, w392) -> (w399:dbl[])
                n282 = Multiply(x=w399, y=w388) -> (x*y=w398:dbl[])
                n283 = Index Array(array=w388, index=0) -> (element=w395:dbl)
                n284 = Add Array Elements(numeric array=w398) -> (sum=w397:dbl)
                n285 = In Range and Coerce(upper limit=0.55, x=w397, lower limit=-0.55) -> (coerced(x)=w409:dbl)  [unwired: 1 out]
                n286 = Subtract(x=w409, y=w397) -> (x-y=w408:dbl)
                n287 = Reciprocal(x=w395) -> (1/x=w407:dbl)
                n288 = disable-structure shown="Enabled" {
                  disable-tunnel: w409 -> [w445 w454]
                  disable-tunnel: [w444 w454] -> w406
                  frame Enabled {
                    n289 = flat-sequence {
                      tunnel: w445 -> [w453]
                      tunnel: [w447] -> w444
                      frame #0 {
                        n290 = Multiply(x=w453, y="lpf gain") -> (x*y=w451:dbl)
                        n291 = Decrement(x="lpf gain") -> (x-1=w452:dbl)
                        n292 = feedback #10(0.0) -> (w449:dbl)
                        n293 = Multiply(x=w452, y=w449) -> (x*y=w450:dbl)
                        n294 = Subtract(x=w451, y=w450) -> (x-y=w447:dbl)
                        n295 = feedback-in #10(w447) -> ()
                      }
                    }
                  }
                  frame Disabled {
                  }
                }
                n296 = Multiply(x=w408, y=w407) -> (x*y=w413:dbl)
                n297 = feedback-in #9(w413) -> ()
              }
            }
            n298 = Select(t=w346, s="Steer input", f="Manual Steering torque") -> (s? t:f=w348:dbl)
            "Waveform Chart 3" <- w348
            n299 = global write "rio_Global.vi" "steering torque"(w348) -> ()
          }
          frame #5 {
            n300 = Get Date/Time In Seconds() -> (seconds since 1Jan1904=w480:timestamp)
            n301 = global read "rio_Global.vi" "LCM_CON_T 2"() -> (w489:T6)
            n302 = To Double Precision Float(number=w480) -> (double precision float=w479:dbl)
            n303 = Unbundle By Name(w489) -> ("hash"=w490:i64)
            n304 = Multiply(x=w479, y=1000000.0) -> (x*y=w483:dbl)
            n305 = global read "rio_Global.vi" "PWM Brake"() -> (w466:dbl)
            n306 = global read "rio_Global.vi" "Ref_str_ang"() -> (w469:dbl)
            n307 = global read "rio_Global.vi" "PWM GAS"() -> (w465:dbl)
            n308 = global read "rio_Global.vi" "Solenoid"() -> (w473:bool)
            n309 = local read "Ref_VS"() -> (w470:dbl)
            n310 = String To IP(1:"192.168.100.200") -> (0:w474:u32)
            n311 = call "hash.vi"("input"=w490) -> ("output"=w488:i64)  [unwired: 10 in]
            n312 = To Quad Integer(1:w483) -> (0:w481:i64)
            n313 = global read "rio_Global.vi" "Auto"() -> (w476:bool)
            n314 = global read "rio_Global.vi" "Run"() -> (w475:bool)
            n315 = Bundle By Name(cluster=w489, "hash"=w488, "sys time"=w481, "Auto"=w476, "Run"=w475, "Solenoid"=w473, "T lim"=FALSE, "brk_enc"=u8 0, "B PWM"=w466, "T PWM"=w465, "ref_vel"=w470, "ref_bkr_enc"=0.0, "ref_apv"=0.0, "ref_steer"=w469, "net address"=w474) -> (w478:T6)
            n316 = Flatten To String(anything=w478, prepend array or string size? (T)=FALSE) -> (data string=w485:string)  [unwired: 2 in, 2 out]
            n317 = global read "rio_Global.vi" "LCM"() -> (w487:T3)
            n318 = call "LCM_send.vi"("DATA"=w485, "ID"="CON_T", "LCM"=w487) -> ()  [unwired: 7 in, 2 out]
          }
        }
      }
    }
  }
  n319 = flat-sequence {
    frame #0 {
      n320 = for {
        N: 257 -> [_]
        tunnel: [w497] -> w495 mode=indexing
        i -> [w497]
      }
      n321 = Multiply(x=w495, y=0.5) -> (x*y=w493:dbl[])
      "x_view" <- w493
      n322 = Array Subset(array=w493, index=30) -> (w491:dbl[])  [unwired: 1 in]
      n323 = global write "rio_Global.vi" "x_view"(w491) -> ()
    }
    frame #1 {
      n324 = while {
        stop <- FALSE stop-if-true
        n325 = flat-sequence {
          frame #0 {
            n326 = Wait Until Next ms Multiple(millisecond multiple=u32 33) -> ()  [unwired: 1 out]
          }
          frame #1 {
            n327 = local read "x_view"() -> (w500:dbl[])
            n328 = call "mobileye_disp.vi"("x_view"=w500) -> ("XY Graph"=→"XY Graph":cluster{"Y":dbl[], "Y":dbl[]}[])  [unwired: 10 in]
          }
        }
      }
    }
  }
  n329 = flat-sequence {
    frame #0 {
      w503 = u16 7668 ("port")
      w512 = u16 7667 ("port")
      n330 = disable-structure shown="Enabled" {
        frame Disabled {
        }
        frame Enabled {
          w520 = "Avante" ("Car_name")
          w526 = 0.0 ("Ref_str_ang")
          w527 = 1000.0 ("PWM GAS")
          w525 = FALSE ("Auto SW")
          n331 = global write "rio_Global.vi" "Shift control"(0.0 ("Shift control")) -> ()
          n332 = global write "rio_Global.vi" "steering torque"(0.0 ("steering")) -> ()
          n333 = global write "rio_Global.vi" "Solenoid"(FALSE ("CAN A 1")) -> ()
          n334 = global write "rio_Global.vi" "PWM GAS"(w527) -> ()
          n335 = global write "rio_Global.vi" "PWM Brake"(w527) -> ()
          n336 = global write "rio_Global.vi" "Ref_VS"(w526) -> ()
          n337 = global write "rio_Global.vi" "Ref_str_ang"(w526) -> ()
          n338 = global write "rio_Global.vi" "Auto"(w525) -> ()
          n339 = global write "rio_Global.vi" "Car_name"(w520) -> ()
          n340 = call "car_spec.vi"("Car_name"=w520) -> ("turn radius"=w524:dbl, "wheel base"=w523:dbl, "ratio"=w522:dbl, "overall width"=w521:dbl)  [unwired: 5 in, 2 out]
          n341 = global write "rio_Global.vi" "Auto SW"(w525) -> ()
          n342 = global write "rio_Global.vi" "ratio"(w522) -> ()
          n343 = global write "rio_Global.vi" "overall width"(w521) -> ()
          n344 = global write "rio_Global.vi" "wheel base"(w523) -> ()
          n345 = global write "rio_Global.vi" "turn radius"(w524) -> ()
        }
      }
      n346 = xnode "Open FPGA VI Reference"() -> ("FPGA VI Reference Out"=w514:refnum<k20>, "error out"=w515:errorcluster)  [unwired: 2 in]
      n347 = global read "rio_Global.vi" "LCM PC"() -> (w507:T3)
      n348 = Decrement(x=w512) -> (x-1=w513:u16)
      n349 = UDP Open(11:w503) -> (port=w505:refnum<k16>)  [unwired: 4 in, 2 out]
      n350 = xnode "Invoke Method"("FPGA VI Reference In"=w514, "error in"=w515) -> ("FPGA VI Reference Out"=w516:refnum<k20>, "error out"=w517:errorcluster)
      n351 = Bundle By Name(cluster=w507, "port"=w503, "connection ID"=w505, "net address"=u32 0) -> (w506:T3)
      n352 = UDP Open(11:w513) -> (port=w510:refnum<k16>)  [unwired: 4 in, 2 out]
      n353 = xnode "Invoke Method"("FPGA VI Reference In"=w516, "error in"=w517, "Wait Until Done (F)"=FALSE) -> ("FPGA VI Reference Out"=→"FPGA":refnum<k20>)  [unwired: 1 out]
      n354 = global read "rio_Global.vi" "LCM"() -> (w508:T3)
      n355 = Bundle By Name(cluster=w508, "port"=w512, "connection ID"=w510, "net address"=u32 4294967295) -> (w509:T3)
      n356 = global write "rio_Global.vi" "LCM PC"(w506) -> ()
      n357 = global write "rio_Global.vi" "LCM"(w509) -> ()
    }
    frame #1 {
      n358 = flat-sequence {
        tunnel: [w603] -> w531
        tunnel: w531 -> [w610]
        frame #0 {
          n359 = local read "FPGA"() -> (w604:refnum<k20>)
          n360 = xnode "Invoke Method"("FPGA VI Reference In"=w604, "Number of Elements"=u32 0, "Timeout (ms)"=0) -> ("FPGA VI Reference Out"=w606:refnum<k20>, "Elements Remaining"=w607:u32)  [unwired: 1 in, 2 out]
          n361 = xnode "Invoke Method"("FPGA VI Reference In"=w606, "Number of Elements"=w607, "Timeout (ms)"=0) -> ("FPGA VI Reference Out"=w603:refnum<k20>)  [unwired: 1 in, 3 out]
        }
        frame #1 {
          n362 = while {
            tunnel: w610 -> [w611]
            stop <- FALSE stop-if-true
            n363 = flat-sequence {
              tunnel: [w614] -> w612
              tunnel: w611 -> [w614]
              tunnel: w612 -> [w621]
              frame #0 {
                n364 = Wait Until Next ms Multiple(millisecond multiple=u32 50) -> (millisecond timer value=w616:u32)
                n365 = feedback #11(w616) -> (w617:u32)
                n366 = feedback-in #11(w616) -> ()
                n367 = Subtract(x=w616, y=w617) -> (x-y=→"Mobileye_time 50":u32)
              }
              frame #1 {
                n368 = while {
                  tunnel: w621 -> [w667]
                  tunnel: [w664] -> w620 mode=indexing
                  stop <- w662 stop-if-true
                  n369 = xnode "Invoke Method"("FPGA VI Reference In"=w667, "Number of Elements"=u32 16, "Timeout (ms)"=0) -> ("FPGA VI Reference Out"=w663:refnum<k20>, "Data"=w664:u8[], "Elements Remaining"=w661:u32)  [unwired: 1 in, 1 out]
                  n370 = Equal To 0?(x=w661) -> (x = 0?=w662:bool)
                  n371 = Quotient & Remainder(x=w661, y=u32 16) -> (x-y*floor(x/y)=w659:u32)  [unwired: 1 out]
                  n372 = case shown="1, Default" w659 {
                    selector: w659 -> [w670 _]
                    tunnel: w663 -> [w669 _]
                    frame 1, Default {
                      n373 = xnode "Invoke Method"("FPGA VI Reference In"=w669, "Number of Elements"=w670, "Timeout (ms)"=0) -> ()  [unwired: 1 in, 4 out]
                    }
                    frame 0 {
                    }
                  }
                }
                n374 = Empty Array?(array=w620) -> (empty?=w619:bool)
                n375 = case shown="False" w619 {
                  tunnel: w620 -> [w623 _]
                  frame False {
                    n376 = flat-sequence {
                      tunnel: w623 -> [w624]
                      tunnel: [w624] -> w622
                      tunnel: w622 -> [w643]
                      frame #0 {
                        n377 = for {
                          tunnel: w624 -> [w634] mode=indexing
                          w637 = 4 ("length")
                          w635 = 8 ("index")
                          n378 = Delete From Array(array=w634, length=w635, index=w635) -> (deleted portion=w625:u8[], array with subset deleted=w636:u8[])
                          n379 = Delete From Array(array=w636, length=w637, index=w637) -> (deleted portion=w641:u8[], array with subset deleted=w638:u8[])
                          n380 = Type Cast(type=u32 0, x=w638) -> (*(type *) &x=w626:u32)
                          n381 = Type Cast(type=u32 0, x=w641) -> (*(type *) &x=w627:u32)
                          n382 = Multiply(x=w627, y=1e-07) -> (x*y=w632:dbl)
                          n383 = To Time Stamp(1:w632) -> (0:w630:timestamp)
                          n384 = Bundle By Name(cluster=T7 {"identifier"=0, "timestamp"=timestamp(0 s since 1904-01-01), "payload"=[]} ("can cluster"), "identifier"=w626, "payload"=w625, "timestamp"=w630) -> (w628:T7)
                          n385 = call "mobileye_decoder.vi"("can cluster"=w628, "name"="Mobileye560") -> ()  [unwired: 10 in]
                        }
                      }
                      frame #1 {
                        n386 = Array Size(array=w643) -> (size(s)=w644:i32[])
                        n387 = Multiply Array Elements(1:w644) -> (0:w653:i32)
                        n388 = Get Date/Time In Seconds() -> (seconds since 1Jan1904=w649:timestamp)
                        n389 = To Double Precision Float(number=w649) -> (double precision float=w650:dbl)
                        n390 = Reshape Array(w643, w653) -> (w654:u8[])
                        n391 = global read "rio_Global.vi" "LCM_CAN_RAW_SNAP"() -> (w647:T9)
                        n392 = Unbundle By Name(w647) -> ("hash"=w652:i64)
                        n393 = Multiply(x=w650, y=1000000.0) -> (x*y=w648:dbl)
                        n394 = To Quad Integer(1:w648) -> (0:w645:i64)
                        n395 = call "hash.vi"("input"=w652) -> ("output"=w646:i64)  [unwired: 10 in]
                        n396 = Bundle(cluster=w647, "hash"=w646, "sys time"=w645, "size"=w653, "data"=w654) -> (w656:T9)
                        n397 = Flatten To String(anything=w656, prepend array or string size? (T)=FALSE) -> (data string=w658:string)  [unwired: 2 in, 2 out]
                        n398 = global read "rio_Global.vi" "LCM"() -> (w657:T3)
                        n399 = call "LCM_send.vi"("DATA"=w658, "ID"="Mobileye560" ("name"), "LCM"=w657) -> ()  [unwired: 7 in, 2 out]
                      }
                    }
                  }
                  frame True {
                  }
                }
              }
            }
          }
        }
      }
      n400 = flat-sequence {
        tunnel: [w671] -> w530
        tunnel: w530 -> [w712]
        frame #0 {
          n401 = global read "rio_Global.vi" "Car_name"() -> (w673:string)
          n402 = local read "FPGA"() -> (w672:refnum<k20>)
          n403 = case shown="Default" w673 {
            tunnel: w672 -> [w674 w680]
            tunnel: [w674 w675] -> w671
            frame "Prius" {
            }
            frame Default {
              n404 = xnode "Invoke Method"("FPGA VI Reference In"=w680, "Number of Elements"=u32 0, "Timeout (ms)"=0) -> ("FPGA VI Reference Out"=w682:refnum<k20>, "Elements Remaining"=w681:u32)  [unwired: 1 in, 2 out]
              n405 = xnode "Invoke Method"("FPGA VI Reference In"=w682, "Number of Elements"=w681, "Timeout (ms)"=0) -> ("FPGA VI Reference Out"=w678:refnum<k20>)  [unwired: 1 in, 3 out]
              n406 = flat-sequence {
                tunnel: [w693] -> w679
                tunnel: w678 -> [w693]
                frame #0 {
                  n407 = Wait (ms)(milliseconds to wait=u32 100) -> ()  [unwired: 1 out]
                }
              }
              n408 = xnode "Read/Write Control"("FPGA VI Reference In"=w679, "send can 1"=TRUE) -> ("FPGA VI Reference Out"=w688:refnum<k20>)  [unwired: 1 in, 1 out]
              n409 = for {
                N: 100 -> [_]
                tunnel: w688 -> [w696]
                tunnel: [w698] -> w676
                i -> [w695]
                n410 = Split Number(x=u16 65535 ("y")) -> (hi(x)=w707:u8, lo(x)=w706:u8)
                n411 = To Unsigned Byte Integer(number=w695) -> (unsigned 8bit integer=w694:u8)
                n412 = Build Array(u8 0 ("Con steer status"), w706, w707, u8 0 ("element"), w694, u8 0 ("element"), u8 0 ("element")) -> (w701:u8[])
                n413 = Add Array Elements(numeric array=w701) -> (sum=w702:u8)
                n414 = Build Array (concatenate)(w701, w702) -> (w699:u8[])
                n415 = Bundle By Name(cluster=T8 {"timestamp high"=0, "timestamp low"=0, "identifier"=0, "type"=enum."Data Frame", "info A"=0, "info B"=0, "data length"=8, "data"=[0, 0, 0, 0, 0, 0, 0, 0]} ("Mod4/CAN1 input"), "identifier"=u32 912, "data"=w699, "data length"=u8 8) -> (w708:T8)
                n416 = xnode "Read/Write Control"("FPGA VI Reference In"=w696, "Mod2/CAN1 input"=w708) -> ("FPGA VI Reference Out"=w698:refnum<k20>)  [unwired: 1 in, 1 out]
              }
              n417 = flat-sequence {
                tunnel: [w691] -> w677
                tunnel: w676 -> [w691]
                frame #0 {
                  n418 = Wait (ms)(milliseconds to wait=u32 100) -> ()  [unwired: 1 out]
                }
              }
              n419 = xnode "Read/Write Control"("FPGA VI Reference In"=w677, "send can 1"=FALSE) -> ("FPGA VI Reference Out"=w675:refnum<k20>)  [unwired: 1 in, 1 out]
            }
          }
        }
        frame #1 {
          n420 = while {
            tunnel: w712 -> [w713]
            stop <- FALSE stop-if-true
            n421 = flat-sequence {
              tunnel: [w716] -> w714
              tunnel: w713 -> [w716]
              tunnel: w714 -> [w723]
              frame #0 {
                n422 = Wait Until Next ms Multiple(millisecond multiple=u32 10) -> (millisecond timer value=w719:u32)
                n423 = feedback #12(w719) -> (w718:u32)
                n424 = feedback-in #12(w719) -> ()
                n425 = Subtract(x=w719, y=w718) -> (x-y=→"CAN_time 10":u32)
              }
              frame #1 {
                n426 = while {
                  tunnel: w723 -> [w784]
                  tunnel: [w781] -> w722 mode=indexing
                  stop <- w780 stop-if-true
                  n427 = xnode "Invoke Method"("FPGA VI Reference In"=w784, "Number of Elements"=u32 16, "Timeout (ms)"=0) -> ("FPGA VI Reference Out"=w779:refnum<k20>, "Data"=w781:u8[], "Elements Remaining"=w776:u32)  [unwired: 1 in, 1 out]
                  n428 = Equal To 0?(x=w776) -> (x = 0?=w780:bool)
                  n429 = Quotient & Remainder(x=w776, y=u32 16) -> (x-y*floor(x/y)=w777:u32)  [unwired: 1 out]
                  n430 = case shown="1, Default" w777 {
                    selector: w777 -> [w787 _]
                    tunnel: w779 -> [w786 _]
                    frame 1, Default {
                      n431 = xnode "Invoke Method"("FPGA VI Reference In"=w786, "Number of Elements"=w787, "Timeout (ms)"=0) -> ()  [unwired: 1 in, 4 out]
                    }
                    frame 0 {
                    }
                  }
                }
                n432 = Empty Array?(array=w722) -> (empty?=w721:bool)
                n433 = case shown="False" w721 {
                  tunnel: w722 -> [w726 _]
                  frame False {
                    n434 = flat-sequence {
                      tunnel: w726 -> [w727]
                      tunnel: [w727] -> w725
                      tunnel: w725 -> [w760]
                      tunnel: [w745] -> w724
                      tunnel: w724 -> [w768]
                      frame #0 {
                        n435 = for {
                          tunnel: w727 -> [w737] mode=indexing
                          w740 = 4 ("length")
                          w738 = 8 ("index")
                          n436 = Delete From Array(array=w737, length=w738, index=w738) -> (deleted portion=w729:u8[], array with subset deleted=w739:u8[])
                          n437 = Delete From Array(array=w739, length=w740, index=w740) -> (deleted portion=w744:u8[], array with subset deleted=w741:u8[])
                          n438 = Type Cast(type=u32 0, x=w741) -> (*(type *) &x=w730:u32)
                          n439 = Type Cast(type=u32 0, x=w744) -> (*(type *) &x=w731:u32)
                          n440 = Multiply(x=w731, y=1e-07) -> (x*y=w734:dbl)
                          n441 = To Time Stamp(1:w734) -> (0:w733:timestamp)
                          n442 = Bundle By Name(cluster=T7 {"identifier"=0, "timestamp"=timestamp(0 s since 1904-01-01), "payload"=[]} ("can cluster"), "identifier"=w730, "payload"=w729, "timestamp"=w733) -> (w736:T7)
                          n443 = global read "rio_Global.vi" "Car_name"() -> (w728:string)
                          n444 = call "can decoder.vi"("can cluster"=w736, "name"=w728) -> ()  [unwired: 10 in]
                        }
                      }
                      frame #1 {
                        n445 = Array Size(array=w760) -> (size(s)=w761:i32[])
                        n446 = global read "rio_Global.vi" "LCM_CAN_RAW_SNAP"() -> (w758:T9)
                        n447 = Multiply Array Elements(1:w761) -> (0:w752:i32)
                        n448 = Get Date/Time In Seconds() -> (seconds since 1Jan1904=w756:timestamp)
                        n449 = To Double Precision Float(number=w756) -> (double precision float=w755:dbl)
                        n450 = Reshape Array(w760, w752) -> (w751:u8[])
                        n451 = Unbundle By Name(w758) -> ("hash"=w753:i64)
                        n452 = Multiply(x=w755, y=1000000.0) -> (x*y=w757:dbl)
                        n453 = call "hash.vi"("input"=w753) -> ("output"=w759:i64)  [unwired: 10 in]
                        n454 = To Quad Integer(1:w757) -> (0:w745:i64)
                        n455 = Bundle(cluster=w758, "hash"=w759, "sys time"=w745, "size"=w752, "data"=w751) -> (w749:T9)
                        n456 = global read "rio_Global.vi" "Car_name"() -> (w746:string)
                        n457 = Flatten To String(anything=w749, prepend array or string size? (T)=FALSE) -> (data string=w747:string)  [unwired: 2 in, 2 out]
                        n458 = global read "rio_Global.vi" "LCM"() -> (w748:T3)
                        n459 = call "LCM_send.vi"("DATA"=w747, "ID"=w746, "LCM"=w748) -> ()  [unwired: 7 in, 2 out]
                      }
                      frame #2 {
                        n460 = global read "rio_Global.vi" "LCM_CAN_T"() -> (w774:T10)
                        n461 = global read "rio_Global.vi" "C_time"() -> (w770:u32)
                        n462 = global read "rio_Global.vi" "C_mdps str_ang"() -> (w772:dbl)
                        n463 = global read "rio_Global.vi" "C_mdps torque"() -> (w762:dbl)
                        n464 = Unbundle By Name(w774) -> ("hash"=w775:i64)
                        n465 = global read "rio_Global.vi" "C_VS_CAN"() -> (w771:dbl)
                        n466 = call "hash.vi"("input"=w775) -> ("output"=w773:i64)  [unwired: 10 in]
                        n467 = To Double Precision Float(number=w770) -> (double precision float=w769:dbl)
                        n468 = Bundle By Name(cluster=w774, "hash"=w773, "mdps str_ang"=w772, "time"=w769, "VS_CAN"=w771, "sys time"=w768, "mdps torque"=w762) -> (w765:T10)
                        n469 = Flatten To String(anything=w765, prepend array or string size? (T)=FALSE) -> (data string=w764:string)  [unwired: 2 in, 2 out]
                        n470 = global read "rio_Global.vi" "LCM"() -> (w767:T3)
                        n471 = call "LCM_send.vi"("DATA"=w764, "ID"="CAN_T", "LCM"=w767) -> ()  [unwired: 7 in, 2 out]
                      }
                    }
                  }
                  frame True {
                  }
                }
              }
            }
          }
        }
      }
      n472 = while {
        stop <- FALSE stop-if-true
        n473 = flat-sequence {
          tunnel: [w538] -> w532
          tunnel: w532 -> [w569]
          frame #0 {
            n474 = Wait Until Next ms Multiple(millisecond multiple=u32 10) -> ()  [unwired: 1 out]
          }
          frame #1 {
            n475 = global read "rio_Global.vi" "Car_name"() -> (w535:string)
            n476 = local read "FPGA"() -> (w540:refnum<k20>)
            n477 = case shown="Default" w535 {
              tunnel: w540 -> [w543 w550]
              tunnel: [_ w548] -> w539
              tunnel: [w543 w546] -> w538
              tunnel: [w542 w545] -> w537
              tunnel: [w541 w544] -> w536
              frame "Prius", "Santafe" {
                n478 = global read "rio_Global.vi" "Auto"() -> (w542:bool)
                n479 = global read "rio_Global.vi" "Run"() -> (w541:bool)
              }
              frame Default {
                n480 = xnode "Read/Write Control"("FPGA VI Reference In"=w550) -> ("FPGA VI Reference Out"=w546:refnum<k20>, "Auto"=w545:bool, "Run"=w549:bool)  [unwired: 1 in, 1 out]
                n481 = global write "rio_Global.vi" "Auto"(w545) -> ()
                n482 = And(x=w545, y=w549) -> (x .and. y?=w544:bool)
                n483 = global write "rio_Global.vi" "Run"(w544) -> ()
                n484 = Not(x=w544) -> (.not. x?=w547:bool)
                n485 = And(x=w545, y=w547) -> (x .and. y?=w548:bool)
              }
            }
            "E - STOP" <- w539
            "Auto" <- w537
            "Run" <- w536
          }
          frame #2 {
            w556 = fxp<+/-,20,5> 0.0 ("Mod3/AO3")
            w562 = fxp<+/-,20,5> 0.0 ("Mod3/AO3")
            n486 = global read "rio_Global.vi" "Car_name"() -> (w555:string)
            n487 = global read "rio_Global.vi" "Auto"() -> (w553:bool)
            n488 = case shown="\"Prius\"" w555 {
              tunnel: [_ w571] -> w560
              tunnel: [_ w570] -> w558
              frame Default {
              }
              frame "Prius" {
                n489 = global read "rio_Global.vi" "Shift control"() -> (w572:dbl)
                n490 = global read "rio_Global.vi" "C_VS_CAN"() -> (w575:dbl)
                n491 = Equal To 0?(x=w575) -> (x = 0?=w577:bool)
                n492 = Not Equal To 0?(x=w572) -> (x != 0?=w576:bool)
                n493 = global read "rio_Global.vi" "Auto"() -> (w574:bool)
                n494 = Compound Arithmetic op=AND(w577, w574, w576) -> (w573:bool)
                n495 = case shown="True" w573 {
                  tunnel: w572 -> [_ w579]
                  tunnel: [_ w579] -> w571
                  tunnel: [_ 5.0] -> w570
                  frame False {
                  }
                  frame True {
                  }
                }
              }
            }
            n496 = global read "rio_Global.vi" "Auto"() -> (w561:bool)
            n497 = And(x="speed control", y=w553) -> (x .and. y?=w552:bool)
            n498 = case shown="True" w552 {
              tunnel: [w587 w600] -> w568
              tunnel: [w587 w599] -> w551
              tunnel: [_ w594] -> w567
              frame False {
                w587 = u16 1000
              }
              frame True {
                n499 = global read "rio_Global.vi" "PWM Brake"() -> (w593:dbl)
                n500 = global read "rio_Global.vi" "PWM GAS"() -> (w602:dbl)
                n501 = Round To Nearest(number=w602) -> (nearest integer value=w597:dbl)
                n502 = Round To Nearest(number=w593) -> (nearest integer value=w592:dbl)
                n503 = global read "rio_Global.vi" "Run"() -> (w590:bool)
                n504 = global read "rio_Global.vi" "Run"() -> (w591:bool)
                n505 = global read "rio_Global.vi" "Solenoid"() -> (w596:bool)
                n506 = Select(t=w597, s=w590, f=1000.0) -> (s? t:f=w595:dbl)
                n507 = Select(t=w592, s=w591, f=1900.0 ("t")) -> (s? t:f=w588:dbl)
                n508 = global read "rio_Global.vi" "Run"() -> (w589:bool)
                n509 = To Unsigned Word Integer(number=w595) -> (unsigned 16bit integer=w600:u16)
                n510 = To Unsigned Word Integer(number=w588) -> (unsigned 16bit integer=w599:u16)
                n511 = Select(t=w596, s=w589, f=w589) -> (s? t:f=w594:bool)
              }
            }
            n512 = case shown="True" w561 {
              tunnel: [_ w581] -> w566
              tunnel: [_ w580] -> w565
              frame False {
              }
              frame True {
                n513 = global read "rio_Global.vi" "steering torque"() -> (w582:dbl)
                n514 = Greater Than 0?(x=w582) -> (x > 0?=w583:bool)
                n515 = case shown="True" w583 {
                  tunnel: w582 -> [w585 w586]
                  tunnel: [w584 _] -> w581
                  tunnel: [_ w586] -> w580
                  frame False {
                    n516 = Absolute Value(x=w585) -> (abs(x)=w584:dbl)
                  }
                  frame True {
                  }
                }
              }
            }
            n517 = To Fixed-Point(fixed-point type=w562, number=w566) -> (fixed-point=w564:fxp<+/-,20,5>)
            n518 = To Fixed-Point(fixed-point type=w562, number=w565) -> (fixed-point=w563:fxp<+/-,20,5>)
            n519 = To Fixed-Point(fixed-point type=w556, number=w558) -> (fixed-point=w557:fxp<+/-,20,5>)
            n520 = To Fixed-Point(fixed-point type=w556, number=w560) -> (fixed-point=w559:fxp<+/-,20,5>)
            n521 = xnode "Read/Write Control"("FPGA VI Reference In"=w569, "Solenoid"=w567, "PWM Gas"=w568, "PWM Brake"=w551, "Mod3/AO0"=w564, "Mod3/AO1"=w563, "Mod3/AO2"=w557, "Mod3/AO3"=w559) -> ()  [unwired: 1 in, 2 out]
          }
        }
      }
    }
  }
  n522 = flat-sequence {
    tunnel: [dbl[] [0.0, 0.0, 0.0, 0.0, 0.0] ("pos(i)")] -> w1
    tunnel: w1 -> [w796]
    frame #0 {
      w792 = FALSE ("get heading")
      w793 = u64 1
      w790 = 0.0 ("dh_hat")
      n523 = local write "GPS init"(w792) -> ()
      n524 = call "getecefdcmref.vi"("map name"=T1."KAIST") -> ("XYZ"=w788:dbl[])  [unwired: 10 in, 4 out]
      n525 = local write "ecef ref"(w788) -> ()
      "vgain" <- 1.0 ("initH")
      "vcount" <- w793
      "hbias" <- w790
      "hcount" <- w793
      "get heading" <- w792
      "get position" <- w792
      "heading error" <- w790
      "h_gps" <- w790
      "rt" <- w790
      "pos error" <- w790
      "POS init" <- TRUE ("POS init")
    }
    frame #1 {
      (unwired) FALSE
      n526 = while {
        shift-right: [w900] -> _
        shift-left: w796 -> [w901]
        stop <- FALSE stop-if-true
        n527 = flat-sequence {
          tunnel: [w932] -> w904
          tunnel: w901 -> [w932]
          tunnel: w904 -> [w935]
          tunnel: [w934] -> w903
          tunnel: [w934] -> w902
          tunnel: [w1349] -> w900
          tunnel: w903 -> [w1350]
          tunnel: w902 -> [w1349]
          frame #0 {
            n528 = global read "rio_Global.vi" "C_ts"() -> (→"dt":dbl)
            n529 = global read "rio_Global.vi" "C_WHL_SPD_RR"() -> (w918:dbl)
            n530 = global read "rio_Global.vi" "C_WHL_SPD_RL"() -> (w917:dbl)
            n531 = Wait Until Next ms Multiple(millisecond multiple=u32 10) -> (millisecond timer value=w930:u32)
            n532 = feedback #13(w930) -> (w929:u32)
            n533 = feedback-in #13(w930) -> ()
            n534 = Subtract(x=w930, y=w929) -> (x-y=w928:u32)
            n535 = Subtract(x=w918, y=w917) -> (x-y=w925:dbl)
            n536 = global read "rio_Global.vi" "overall width"() -> (w909:dbl)
            n537 = To Long Integer(number=w928) -> (32bit integer=→"Pos_time 10":i32)
            n538 = Divide(x=w925, y=3.6) -> (x/y=w923:dbl)
            n539 = Divide(x=w923, y=w909) -> (x/y=w922:dbl)
            n540 = global read "rio_Global.vi" "C_VS_CAN"() -> (w911:dbl)
            n541 = global read "rio_Global.vi" "C_yaw_rate"() -> (w908:dbl)
            n542 = Multiply(x=w922, y=180.0) -> (x*y=w920:dbl)
            n543 = Sign(1:w911) -> (0:w910:dbl)
            n544 = Divide(x=w920, y=3.141592653589793) -> (x/y=w914:dbl)
            n545 = Compound Arithmetic op=MULTIPLY(w914, 1.2144 ("scale"), w910) -> (w912:dbl)
            n546 = Multiply(x=w908, y=1.0) -> (x*y=w907:dbl)
            n547 = Select(t=w912, s=FALSE, f=w907) -> (s? t:f=→"C_yaw_rate":dbl)
          }
          frame #1 {
            n548 = flat-sequence {
              tunnel: w935 -> [w942]
              tunnel: [w942] -> w933
              tunnel: [w1065] -> w934
              tunnel: w933 -> [w1066]
              frame #0 {
                n549 = disable-structure shown="Enabled" {
                  disable-tunnel: [w962 w963] -> w937
                  disable-tunnel: [w943 w964] -> w936
                  frame Disabled {
                    n550 = global read "rio_Global.vi" "gps_pos 1"() -> (w959:dbl[])
                    n551 = global read "rio_Global.vi" "gps_pos 2"() -> (w946:dbl[])
                    n552 = Add(x=w959, y=w946) -> (x+y=w961:dbl[])
                    n553 = Index Array(array=w959, index #1=0 ("index")) -> (element #1=w958:dbl, element #2=w957:dbl)  [unwired: 1 in]
                    n554 = Index Array(array=w946, index #1=0 ("index")) -> (element #1=w947:dbl, element #2=w948:dbl)  [unwired: 1 in]
                    n555 = feedback #14(w958) -> (w956:dbl)
                    n556 = feedback-in #14(w958) -> ()
                    n557 = feedback #15(w947) -> (w949:dbl)
                    n558 = feedback-in #15(w947) -> ()
                    n559 = Not Equal?(x=w958, y=w956) -> (x != y?=w955:bool)
                    n560 = Not Equal?(x=w947, y=w949) -> (x != y?=w950:bool)
                    n561 = Not Equal To 0?(x=w957) -> (x != 0?=w954:bool)
                    n562 = Not Equal To 0?(x=w948) -> (x != 0?=w951:bool)
                    n563 = And(x=w955, y=w954) -> (x .and. y?=w944:bool)
                    n564 = And(x=w950, y=w951) -> (x .and. y?=w945:bool)
                    n565 = And(x=w944, y=w945) -> (x .and. y?=w962:bool)
                    n566 = Multiply(x=w961, y=0.5) -> (x*y=w943:dbl[])
                  }
                  frame Enabled {
                    n567 = global read "rio_Global.vi" "gps_pos 1"() -> (w964:dbl[])
                    n568 = Index Array(array=w964, index #1=0 ("index")) -> (element #1=w970:dbl, element #2=w969:dbl)  [unwired: 1 in]
                    n569 = feedback #16(w970) -> (w968:dbl)
                    n570 = feedback-in #16(w970) -> ()
                    n571 = Not Equal?(x=w970, y=w968) -> (x != y?=w967:bool)
                    n572 = Not Equal To 0?(x=w969) -> (x != 0?=w966:bool)
                    n573 = And(x=w967, y=w966) -> (x .and. y?=w963:bool)
                  }
                }
                "pos_gps" <- w936
                n574 = disable-structure shown="Enabled" {
                  disable-tunnel: [w1016 w1047] -> w941
                  disable-tunnel: [w1015 w1026] -> w940
                  disable-tunnel: [w987 w1037] -> w939
                  disable-tunnel: [w975 w1032] -> w938
                  frame Disabled {
                    n575 = global read "rio_Global.vi" "gps_vel 1"() -> (w1014:dbl[])
                    n576 = global read "rio_Global.vi" "gps_vel 2"() -> (w993:dbl[])
                    n577 = Index Array(array=w1014, index #1=0 ("index"), index #2=1 ("index"), index #3=4 ("index"), index #4=2 ("index")) -> (element #1=w1005:dbl, element #2=w1010:dbl, element #3=w1007:dbl, element #4=w979:dbl)
                    n578 = Index Array(array=w993, index #1=0 ("index"), index #2=1 ("index"), index #3=4 ("index"), index #4=2 ("index")) -> (element #1=w1002:dbl, element #2=w997:dbl, element #3=w1000:dbl, element #4=w978:dbl)
                    n579 = global read "rio_Global.vi" "C_VS_CAN"() -> (w972:dbl)
                    n580 = global read "rio_Global.vi" "C_VS_CAN"() -> (w1019:dbl)
                    n581 = Add(x=w979, y=w978) -> (x+y=w977:dbl)
                    n582 = call "angleconv.vi"("deg"=w1007) -> ("rad"=w990:dbl)  [unwired: 9 in, 1 out]
                    n583 = call "angleconv.vi"("deg"=w1000) -> ("rad"=w989:dbl)  [unwired: 9 in, 1 out]
                    n584 = Not Equal To 0?(x=w997) -> (x != 0?=w998:bool)
                    n585 = feedback #17(0.0 ("Real Matrix Element")) -> (w1004:dbl)
                    n586 = feedback-in #17(w1005) -> ()
                    n587 = feedback #18(0.0 ("Real Matrix Element")) -> (w1003:dbl)
                    n588 = feedback-in #18(w1002) -> ()
                    n589 = Not Equal?(x=w1005, y=w1004) -> (x != y?=w1011:bool)
                    n590 = Not Equal?(x=w1002, y=w1003) -> (x != y?=w996:bool)
                    n591 = Greater Or Equal To 0?(x=w1019) -> (x >= 0?=w1020:bool)
                    n592 = Not Equal To 0?(x=w1010) -> (x != 0?=w1009:bool)
                    n593 = Absolute Value(x=w972) -> (abs(x)=w971:dbl)
                    n594 = Multiply(x=w977, y=0.5) -> (x*y=w986:dbl)
                    n595 = call "headingweightsum.vi"("a"=0.5, "h1"=w989, "h2"=w990) -> ("a*h2+(1-a)*h1"=w1018:dbl)  [unwired: 8 in]
                    n596 = And(x=w1011, y=w1009) -> (x .and. y?=w992:bool)
                    n597 = And(x=w996, y=w998) -> (x .and. y?=w991:bool)
                    n598 = Divide(x=w986, y=w971) -> (x/y=w987:dbl)
                    n599 = Select(t=0.0, s=w1020, f=3.141592653589793) -> (s? t:f=w1017:dbl)
                    n600 = Decrement(x=w987) -> (x-1=w983:dbl)
                    n601 = call "headingoperater.vi"("h1"=w1017, "h2"=w1018) -> ("h2-h1"=w1016:dbl)  [unwired: 8 in, 1 out]
                    n602 = And(x=w992, y=w991) -> (x .and. y?=w1015:bool)
                    n603 = Absolute Value(x=w983) -> (abs(x)=w984:dbl)
                    n604 = Greater?(x=w971, y=15.0) -> (0:w973:bool)
                    n605 = Less?(x=w984, y=0.05) -> (x < y?=w976:bool)
                    n606 = Compound Arithmetic op=AND(w973, w976, w1015) -> (w975:bool)
                  }
                  frame Enabled {
                    n607 = global read "rio_Global.vi" "gps_vel 1"() -> (w1046:dbl[])
                    n608 = global read "rio_Global.vi" "C_VS_CAN"() -> (w1030:dbl)
                    n609 = global read "rio_Global.vi" "C_VS_CAN"() -> (w1049:dbl)
                    n610 = Index Array(array=w1046, index #1=0 ("index"), index #2=1 ("index"), index #3=4 ("index"), index #4=2 ("index")) -> (element #1=w1025:dbl, element #2=w1042:dbl, element #3=w1039:dbl, element #4=w1028:dbl)
                    n611 = Greater Or Equal To 0?(x=w1049) -> (x >= 0?=w1050:bool)
                    n612 = Absolute Value(x=w1030) -> (abs(x)=w1029:dbl)
                    n613 = feedback #19(w1025) -> (w1038:dbl)
                    n614 = feedback-in #19(w1025) -> ()
                    n615 = Divide(x=w1028, y=w1029) -> (x/y=w1037:dbl)
                    n616 = call "angleconv.vi"("deg"=w1039) -> ("rad"=w1027:dbl)  [unwired: 9 in, 1 out]
                    n617 = Select(t=0.0, s=w1050, f=3.141592653589793) -> (s? t:f=w1048:dbl)
                    n618 = Not Equal?(x=w1025, y=w1038) -> (x != y?=w1043:bool)
                    n619 = Decrement(x=w1037) -> (x-1=w1034:dbl)
                    n620 = Not Equal To 0?(x=w1042) -> (x != 0?=w1041:bool)
                    n621 = call "headingoperater.vi"("h1"=w1048, "h2"=w1027) -> ("h2-h1"=w1047:dbl)  [unwired: 8 in, 1 out]
                    n622 = And(x=w1043, y=w1041) -> (x .and. y?=w1026:bool)
                    n623 = Absolute Value(x=w1034) -> (abs(x)=w1035:dbl)
                    n624 = Greater?(x=w1029, y=15.0) -> (0:w1023:bool)
                    n625 = Less?(x=w1035, y=0.05) -> (x < y?=w1024:bool)
                    n626 = Compound Arithmetic op=AND(w1026, w1024, w1023) -> (w1032:bool)
                  }
                }
                n627 = local write "get position"(w937) -> ()
                n628 = local write "h_gps"(w941) -> ()
                n629 = case shown="True" w938 {
                  tunnel: w939 -> [_ w1060]
                  frame False {
                  }
                  frame True {
                    w1054 = u64 18446744073709551615
                    n630 = local read "vcount"() -> (w1057:u64)
                    n631 = local read "vgain"() -> (w1062:dbl)
                    n632 = Increment(x=w1057) -> (x+1=w1056:u64)
                    n633 = Multiply(x=w1062, y=w1057) -> (x*y=w1061:dbl)
                    n634 = Not Equal?(x=w1057, y=w1054) -> (x != y?=w1055:bool)
                    n635 = Add(x=w1060, y=w1061) -> (x+y=w1059:dbl)
                    n636 = Select(t=w1056, s=w1055, f=w1054) -> (s? t:f=w1053:u64)
                    n637 = local write "vcount"(w1053) -> ()
                    n638 = Divide(x=w1059, y=w1053) -> (x/y=w1058:dbl)
                    n639 = local write "vgain"(w1058) -> ()
                  }
                }
                n640 = local write "get heading"(w940) -> ()
              }
              frame #1 {
                n641 = local read "dt"() -> (w1064:dbl)
                n642 = Greater Than 0?(x=w1064) -> (x > 0?=w1063:bool)
                n643 = case shown="True" w1063 {
                  tunnel: w1066 -> [w1067 w1070]
                  tunnel: [w1067 w1069] -> w1065
                  frame False {
                  }
                  frame True {
                    n644 = flat-sequence {
                      tunnel: w1070 -> [w1105]
                      tunnel: [w1083] -> w1068
                      tunnel: [w1133] -> w1069
                      tunnel: w1068 -> [w1132]
                      frame #0 {
                        n645 = global read "rio_Global.vi" "C_VS_CAN"() -> (w1073:dbl)
                        n646 = local read "C_yaw_rate"() -> (w1071:dbl)
                        n647 = Equal To 0?(x=w1073) -> (x = 0?=w1075:bool)
                        n648 = case shown="True" w1075 {
                          tunnel: [w1107 _] -> w1074
                          tunnel: w1071 -> [w1106 w1111]
                          frame False {
                            n649 = local read "hbias"() -> (w1110:dbl)
                            n650 = Subtract(x=w1106, y=w1110) -> (x-y=w1108:dbl)
                            n651 = Negate(x=w1108) -> (-x=w1109:dbl)
                            n652 = call "angleconv.vi"("deg"=w1109) -> ("rad"=w1107:dbl)  [unwired: 9 in, 1 out]
                          }
                          frame True {
                            w1114 = u64 18446744073709551615
                            n653 = local read "hcount"() -> (w1117:u64)
                            n654 = local read "hbias"() -> (w1120:dbl)
                            n655 = Increment(x=w1117) -> (x+1=w1116:u64)
                            n656 = Not Equal?(x=w1117, y=w1114) -> (x != y?=w1115:bool)
                            n657 = Multiply(x=w1120, y=w1117) -> (x*y=w1119:dbl)
                            n658 = Add(x=w1111, y=w1119) -> (x+y=w1118:dbl)
                            n659 = Select(t=w1116, s=w1115, f=w1114) -> (s? t:f=w1113:u64)
                            n660 = local write "hcount"(w1113) -> ()
                            n661 = Divide(x=w1118, y=w1113) -> (x/y=w1112:dbl)
                            n662 = local write "hbias"(w1112) -> ()
                          }
                        }
                        n663 = global read "rio_Global.vi" "C_VS_CAN"() -> (w1072:dbl)
                        n664 = local read "vgain"() -> (w1078:dbl)
                        n665 = Multiply(x=w1072, y=w1078) -> (x*y=w1077:dbl)
                        n666 = Divide(x=w1077, y=3.6) -> (x/y=w1076:dbl)
                        n667 = Index Array(array=w1105, index #1=0 ("index"), index #2=3 ("index"), index #3=1 ("index"), index #4=3 ("index")) -> (element #1=w1099:dbl, element #2=w1097:dbl, element #3=w1093:dbl, element #4=w1088:dbl)
                        n668 = local read "dt"() -> (w1102:dbl)
                        n669 = local read "dt"() -> (w1086:dbl)
                        n670 = Multiply(x=w1076, y=w1102) -> (x*y=w1098:dbl)
                        n671 = Multiply(x=w1086, y=w1074) -> (x*y=w1079:dbl)
                        n672 = Cosine(x=w1097) -> (cos(x)=w1103:dbl)
                        n673 = Sine(x=w1097) -> (sin(x)=w1096:dbl)
                        n674 = Multiply(x=w1103, y=w1098) -> (x*y=w1100:dbl)
                        n675 = Multiply(x=w1098, y=w1096) -> (x*y=w1095:dbl)
                        n676 = local write "rt"(w1079) -> ()
                        n677 = Add(x=w1099, y=w1100) -> (x+y=w1092:dbl)
                        n678 = Add(x=w1095, y=w1093) -> (x+y=w1091:dbl)
                        n679 = call "headingoperater.vi"("h1"=w1079, "h2"=w1088) -> ("h2+h1"=w1087:dbl)  [unwired: 8 in, 1 out]
                        n680 = Build Array(w1092, w1091, w1076, w1087, w1074) -> (w1083:dbl[])
                        n681 = Index Array(array=w1083, index=3) -> (element=w1082:dbl)
                        n682 = local read "h_gps"() -> (w1081:dbl)
                        n683 = call "headingoperater.vi"("h1"=w1082, "h2"=w1081) -> ("h2-h1"=w1085:dbl)  [unwired: 8 in, 1 out]
                        n684 = Absolute Value(x=w1085) -> (abs(x)=w1080:dbl)
                        n685 = local write "heading error"(w1080) -> ()
                      }
                      frame #1 {
                        n686 = local read "get heading"() -> (w1140:bool)
                        n687 = local read "get position"() -> (w1139:bool)
                        n688 = local read "POS init"() -> (w1125:bool)
                        n689 = case shown="False" w1125 {
                          tunnel: w1140 -> [w1143 w1150]
                          tunnel: w1139 -> [w1147 w1149]
                          tunnel: [w1141 w1148] -> w1135
                          frame False {
                            n690 = local read "heading error"() -> (w1144:dbl)
                            n691 = Less?(x=w1144, y=0.05) -> (x < y?=w1145:bool)
                            n692 = And(x=w1143, y=w1145) -> (x .and. y?=w1142:bool)
                            n693 = Or(x=w1142, y=w1147) -> (x .or. y?=w1141:bool)
                          }
                          frame True {
                            n694 = disable-structure shown="Enabled" {
                              disable-tunnel: w1150 -> [w1153 w1155]
                              disable-tunnel: w1149 -> [w1152 w1154]
                              disable-tunnel: [w1151 w1156] -> w1148
                              frame Disabled {
                                n695 = And(x=w1153, y=w1152) -> (x .and. y?=w1151:bool)
                              }
                              frame Enabled {
                                n696 = Or(x=w1155, y=w1154) -> (x .or. y?=w1156:bool)
                              }
                            }
                          }
                        }
                        n697 = global read "rio_Global.vi" "C_VS_CAN"() -> (w1138:dbl)
                        n698 = local read "heading error"() -> (w1128:dbl)
                        n699 = Absolute Value(x=w1138) -> (abs(x)=w1137:dbl)
                        n700 = local read "POS init"() -> (w1126:bool)
                        n701 = Greater?(x=w1137, y=5.0) -> (0:w1134:bool)
                        n702 = Less?(x=w1128, y=1.0) -> (x < y?=w1127:bool)
                        n703 = Or(x=w1127, y=w1126) -> (x .or. y?=w1129:bool)
                        n704 = And(x=w1135, y=w1134) -> (x .and. y?=w1130:bool)
                        n705 = And(x=w1130, y=w1129) -> (x .and. y?=w1123:bool)
                        n706 = Select(t=FALSE, s="GPS init", f=w1123) -> (s? t:f=w1122:bool)
                        n707 = case shown="True" w1122 {
                          tunnel: [w1160 w1189] -> w1133
                          tunnel: w1132 -> [w1161 w1192]
                          frame False {
                            n708 = global read "rio_Global.vi" "C_VS_CAN"() -> (w1164:dbl)
                            n709 = local read "POS init"() -> (w1163:bool)
                            n710 = Equal To 0?(x=w1164) -> (x = 0?=w1162:bool)
                            n711 = local read "GPS init"() -> (w1157:bool)
                            n712 = And(x=w1163, y=w1162) -> (x .and. y?=w1159:bool)
                            n713 = Or(x=w1159, y=w1157) -> (x .or. y?=w1158:bool)
                            n714 = case shown="True" w1158 {
                              tunnel: w1161 -> [w1165 w1166]
                              tunnel: [w1165 w1168] -> w1160
                              tunnel: w1157 -> [_ w1167]
                              frame False {
                              }
                              frame True {
                                n715 = case shown="True" w1167 {
                                tunnel: [w1179 w1188] -> w1168
                                tunnel: w1166 -> [w1174 w1182]
                                frame True {
                                n716 = Index Array(array=w1174, index #1=2 ("index")) -> (element #2=w1169:dbl, element #3=w1172:dbl)  [unwired: 2 in, 1 out]
                                n717 = local read "pos_gps"() -> (w1175:dbl[])
                                n718 = local write "GPS init"(FALSE ("GPS init")) -> ()
                                n719 = Index Array(array=w1175, index #1=2 ("index")) -> (element #1=w1177:dbl, element #2=w1176:dbl)  [unwired: 1 in]
                                n720 = local read "h_gps"() -> (w1170:dbl)
                                n721 = Build Array(w1177, w1176, w1169, w1170, w1172) -> (w1179:dbl[])
                                }
                                frame False {
                                w1181 = 0.0 ("element")
                                n722 = Index Array(array=w1182, index=3) -> (element=w1180:dbl)
                                n723 = local read "pos_gps"() -> (w1184:dbl[])
                                n724 = Index Array(array=w1184, index #1=2 ("index")) -> (element #1=w1186:dbl, element #2=w1185:dbl)  [unwired: 1 in]
                                n725 = Build Array(w1186, w1185, w1181, w1180, w1181) -> (w1188:dbl[])
                                }
                                }
                              }
                            }
                          }
                          frame True {
                            n726 = flat-sequence {
                              tunnel: w1192 -> [w1193]
                              tunnel: [w1193] -> w1191
                              tunnel: w1191 -> [w1234]
                              tunnel: [w1234] -> w1190
                              tunnel: w1190 -> [w1261]
                              tunnel: [w1265] -> w1189
                              frame #0 {
                                w1202 = 0.0 ("element")
                                w1206 = 0.0 ("element")
                                w1208 = 0.0 ("element")
                                w1210 = 0.0 ("element")
                                w1212 = 0.0 ("element")
                                n727 = Index Array(array=w1193, index #1=3 ("index"), index #2=2 ("index"), index #3=3 ("index"), index #4=2 ("index")) -> (element #1=w1222:dbl, element #2=w1224:dbl, element #3=w1227:dbl, element #4=w1216:dbl)
                                n728 = Negate(x=w1224) -> (-x=w1223:dbl)
                                n729 = Sine & Cosine(0:w1227) -> (1:w1219:dbl, 2:w1217:dbl)
                                n730 = Multiply(x=w1223, y=w1219) -> (x*y=w1220:dbl)
                                n731 = Multiply(x=w1217, y=w1216) -> (x*y=w1215:dbl)
                                n732 = Cosine(x=w1222) -> (cos(x)=w1221:dbl)
                                n733 = Build Array(w1212, w1212, w1221, w1220, 0.0 ("element")) -> (w1214:dbl[])
                                n734 = Build Array(w1210, w1210, w1219, w1215, 0.0 ("element")) -> (w1213:dbl[])
                                n735 = Build Array(w1208, w1208, w1208, w1208, w1208) -> (w1207:dbl[])
                                n736 = Build Array(w1206, w1206, w1206, w1206, 1.0 ("element")) -> (w1204:dbl[])
                                n737 = Build Array(w1202, w1202, w1202, w1202, w1202) -> (w1203:dbl[])
                                n738 = Build Array(w1214, w1213, w1207, w1204, w1203) -> (w1200:dbl[][])
                                n739 = call-poly <vilib>:"Array To Matrix.vi"("Real 2D Array"=w1200) -> ("Real Matrix"=w1198:T11)
                                n740 = global read "rio_Global.vi" "P"() -> (w1201:T11)
                                n741 = Transpose Matrix(1:w1198) -> (0:w1197:T11)
                                n742 = call-poly <vilib>:"Multiply.vi"("Real Matrix B"=w1201, "Real Matrix A"=w1198) -> ("A * B"=w1199:T11)
                                n743 = call-poly <vilib>:"Multiply.vi"("Real Matrix B"=w1197, "Real Matrix A"=w1199) -> ("A * B"=w1196:T11)
                                n744 = global read "rio_Global.vi" "Q"() -> (w1195:T11)
                                n745 = call-poly <vilib>:"Add.vi"("Real Matrix B"=w1195, "Real Matrix A"=w1196) -> ("A + B"=w1194:T11)
                                n746 = global write "rio_Global.vi" "Pp"(w1194) -> ()
                              }
                              frame #1 {
                                n747 = global read "rio_Global.vi" "Pp"() -> (w1259:T11)
                                n748 = global read "rio_Global.vi" "H"() -> (w1258:T11)
                                n749 = Array Subset(array=w1234, index=0, length=2) -> (w1241:dbl[])
                                n750 = local read "pos_gps"() -> (w1237:dbl[])
                                n751 = call-poly <vilib>:"Multiply.vi"("Real Matrix B"=w1259, "Real Matrix A"=w1258) -> ("A * B"=w1257:T11)
                                n752 = Transpose Matrix(1:w1258) -> (0:w1256:T11)
                                n753 = call-poly <vilib>:"Multiply.vi"("Real Matrix B"=w1256, "Real Matrix A"=w1257) -> ("A * B"=w1255:T11)
                                n754 = Array Subset(array=w1237, index=2, length=2) -> (w1240:dbl[])
                                n755 = Subtract(x=w1240, y=w1241) -> (x-y=w1242:dbl[])
                                n756 = global read "rio_Global.vi" "H"() -> (w1253:T11)
                                n757 = global read "rio_Global.vi" "R"() -> (w1254:T11)
                                n758 = global read "rio_Global.vi" "Pp"() -> (w1252:T11)
                                n759 = call-poly <vilib>:"Add.vi"("Real Matrix B"=w1254, "Real Matrix A"=w1255) -> ("A + B"=w1249:T11)
                                n760 = Square(x=w1242) -> (x^2=w1243:dbl[])
                                n761 = Transpose Matrix(1:w1253) -> (0:w1251:T11)
                                n762 = local read "heading error"() -> (w1246:dbl)
                                n763 = call-poly <vilib>:"Multiply.vi"("Real Matrix B"=w1251, "Real Matrix A"=w1252) -> ("A * B"=w1250:T11)
                                n764 = Add Array Elements(numeric array=w1243) -> (sum=w1244:dbl)
                                n765 = call-poly <vilib>:"Inverse Matrix.vi"("Input Matrix"=w1249) -> ("Inverse Matrix"=w1248:T11)  [unwired: 1 in, 1 out]
                                n766 = call-poly <vilib>:"Multiply.vi"("Real Matrix B"=w1248, "Real Matrix A"=w1250) -> ("A * B"=w1247:T11)
                                n767 = Square Root(x=w1244) -> (sqrt(x)=w1233:dbl)
                                n768 = global write "rio_Global.vi" "K"(w1247) -> ()
                                n769 = Less?(x=w1233, y=2.5) -> (x < y?=w1230:bool)
                                n770 = Less?(x=w1246, y=0.05) -> (x < y?=w1231:bool)
                                n771 = And(x=w1231, y=w1230) -> (x .and. y?=w1229:bool)
                                n772 = case shown="True" w1229 {
                                frame False {
                                }
                                frame True {
                                n773 = local write "POS init"(FALSE ("Kalman init")) -> ()
                                }
                                }
                              }
                              frame #2 {
                                n774 = disable-structure shown="Enabled" {
                                disable-tunnel: [w1283 w1285] -> w1263
                                disable-tunnel: w1261 -> [_ w1294]
                                frame Disabled {
                                n775 = local read "get position"() -> (w1283:bool)
                                }
                                frame Enabled {
                                n776 = Array Subset(array=w1294, index=0, length=2) -> (w1292:dbl[])
                                n777 = local read "pos_gps"() -> (w1297:dbl[])
                                n778 = Array Subset(array=w1297, index=2, length=2) -> (w1293:dbl[])
                                n779 = disable-structure shown="Enabled" {
                                disable-tunnel: [w1300 TRUE ("Kalman init")] -> w1287
                                frame Disabled {
                                n780 = local read "POS init"() -> (w1300:bool)
                                }
                                frame Enabled {
                                }
                                }
                                n781 = Subtract(x=w1293, y=w1292) -> (x-y=w1291:dbl[])
                                n782 = Square(x=w1291) -> (x^2=w1290:dbl[])
                                n783 = Add Array Elements(numeric array=w1290) -> (sum=w1289:dbl)
                                n784 = Square Root(x=w1289) -> (sqrt(x)=w1284:dbl)
                                n785 = local write "pos error"(w1284) -> ()
                                n786 = Less?(x=w1284, y=3.0) -> (x < y?=w1286:bool)
                                n787 = Or(x=w1287, y=w1286) -> (x .or. y?=w1285:bool)
                                }
                                }
                                n788 = disable-structure shown="Enabled" {
                                disable-tunnel: [w1277 w1278] -> w1264
                                frame Disabled {
                                n789 = local read "get heading"() -> (w1277:bool)
                                }
                                frame Enabled {
                                n790 = local read "heading error"() -> (w1281:dbl)
                                n791 = local read "POS init"() -> (w1279:bool)
                                n792 = Less?(x=w1281, y=0.1) -> (x < y?=w1280:bool)
                                n793 = Or(x=w1280, y=w1279) -> (x .or. y?=w1278:bool)
                                }
                                }
                                n794 = Index Array(array=w1261, index=3) -> (element=w1268:dbl)
                                n795 = global read "rio_Global.vi" "K"() -> (w1276:T11)
                                n796 = global read "rio_Global.vi" "H"() -> (w1275:T11)
                                n797 = global read "rio_Global.vi" "Pp"() -> (w1273:T11)
                                n798 = call-poly <vilib>:"Multiply.vi"("Real Matrix B"=w1275, "Real Matrix A"=w1276) -> ("A * B"=w1274:T11)
                                n799 = global read "rio_Global.vi" "Pp"() -> (w1271:T11)
                                n800 = call-poly <vilib>:"Multiply.vi"("Real Matrix B"=w1273, "Real Matrix A"=w1274) -> ("A * B"=w1272:T11)
                                n801 = call-poly <vilib>:"Subtract.vi"("Real Matrix B"=w1272, "Real Matrix A"=w1271) -> ("A - B"=w1270:T11)
                                n802 = global write "rio_Global.vi" "P"(w1270) -> ()
                                n803 = case shown="True" w1264 {
                                tunnel: w1268 -> [w1326 w1333]
                                tunnel: [w1326 w1328] -> w1262
                                frame False {
                                }
                                frame True {
                                n804 = global read "rio_Global.vi" "K"() -> (w1332:T11)
                                n805 = Index Array(array=w1332, index (row)=3, index (col)=2 ("disabled index (col)")) -> (element=w1329:dbl)
                                n806 = local read "h_gps"() -> (w1327:dbl)
                                n807 = call "headingweightsum2.vi"("a"=w1329, "h2"=w1327, "h1"=w1333) -> ("a*h2+(1-a)*h1"=w1328:dbl)  [unwired: 8 in]
                                }
                                }
                                n808 = case shown="True" w1263 {
                                tunnel: w1261 -> [w1302 w1314]
                                tunnel: [w1302 w1313] -> w1267
                                tunnel: w1262 -> [_ w1303]
                                frame False {
                                }
                                frame True {
                                n809 = disable-structure shown="Enabled" {
                                disable-tunnel: [w1324 w1325] -> w1304
                                disable-tunnel: w1303 -> [_ w1325]
                                frame Disabled {
                                n810 = local read "h_gps"() -> (w1324:dbl)
                                }
                                frame Enabled {
                                }
                                }
                                n811 = local read "pos_gps"() -> (w1308:dbl[])
                                n812 = call-poly <vilib>:"Array To Matrix.vi"("Real 1D Array"=w1314) -> ("Real Matrix (Column Vector)"=w1318:T11)
                                n813 = Array Subset(array=w1308, index=2, length=2) -> (w1309:dbl[])
                                n814 = Build Array (concatenate)(w1309, w1304) -> (w1305:dbl[])
                                n815 = global read "rio_Global.vi" "H"() -> (w1323:T11)
                                n816 = call-poly <vilib>:"Multiply.vi"("Real Matrix B"=w1318, "Real Matrix A"=w1323) -> ("A * B"=w1322:T11)
                                n817 = call-poly <vilib>:"Array To Matrix.vi"("Real 1D Array"=w1305) -> ("Real Matrix (Column Vector)"=w1321:T11)
                                n818 = call-poly <vilib>:"Subtract.vi"("Real Matrix B"=w1322, "Real Matrix A"=w1321) -> ("A - B"=w1319:T11)
                                n819 = global read "rio_Global.vi" "K"() -> (w1320:T11)
                                n820 = call-poly <vilib>:"Multiply.vi"("Real Matrix B"=w1319, "Real Matrix A"=w1320) -> ("A * B"=w1312:T11)
                                n821 = call-poly <vilib>:"Multiply.vi"("Real Matrix A"=w1312, "Real Scalar c"=0.5) -> ("c * A"=w1310:T11)
                                n822 = call-poly <vilib>:"Add.vi"("Real Matrix B"=w1318, "Real Matrix A"=w1310) -> ("A + B"=w1317:T11)
                                n823 = call-poly <vilib>:"Matrix To Array.vi"("Real Matrix"=w1317) -> ("Real 2D Array"=w1316:dbl[][])
                                n824 = Index Array(array=w1316, index (col)=0 ("disabled index (col)")) -> (element=w1313:dbl[])  [unwired: 1 in]
                                }
                                }
                                n825 = Replace Array Subset(array=w1267, new element=w1262, index=3) -> (w1265:dbl[])
                              }
                            }
                          }
                        }
                      }
                    }
                  }
                }
              }
            }
          }
          frame #2 {
            n826 = local read "h_gps"() -> (w1339:dbl)
            n827 = local read "dt"() -> (w1336:dbl)
            n828 = Index Array(array=w1350, index=3) -> (element=w1343:dbl)
            n829 = Array Subset(array=w1350, index=0, length=2) -> (→"pos":dbl[])
            n830 = Greater Than 0?(x=w1336) -> (x > 0?=w1335:bool)
            n831 = call "angleconv.vi"("rad"=w1343) -> ("deg"=→"Heading":dbl)  [unwired: 9 in, 1 out]
            n832 = Greater?(x=1.0, y=w1336) -> (0:w1338:bool)
            n833 = call "headingoperater.vi"("h1"=0.0, "h2"=w1339) -> ("h2+h1"=w1340:dbl)  [unwired: 8 in, 1 out]
            n834 = call "angleconv.vi"("rad"=w1340) -> ("deg"=→"H_GPS":dbl)  [unwired: 9 in, 1 out]
            n835 = Compound Arithmetic op=AND(w1338, w1335) -> (w1334:bool)
            n836 = case shown="True" w1334 {
              tunnel: w1350 -> [_ w1351]
              frame False {
              }
              frame True {
                n837 = flat-sequence {
                  tunnel: w1351 -> [w1375]
                  frame #0 {
                    n838 = Get Date/Time In Seconds() -> (seconds since 1Jan1904=w1366:timestamp)
                    n839 = To Double Precision Float(number=w1366) -> (double precision float=w1360:dbl)
                    n840 = global read "rio_Global.vi" "LCM_POS_T"() -> (w1374:T12)
                    n841 = local read "POS init"() -> (w1356:bool)
                    n842 = Unbundle By Name(w1374) -> ("hash"=w1371:i64)
                    n843 = local read "dt"() -> (w1355:dbl)
                    n844 = Multiply(x=w1360, y=1000000.0) -> (x*y=w1358:dbl)
                    n845 = Array To Cluster(array=w1375) -> (cluster=w1373:T13)
                    n846 = Select(t=0.0, s=w1356, f=w1355) -> (s? t:f=w1353:dbl)
                    n847 = call "hash.vi"("input"=w1371) -> ("output"=w1370:i64)  [unwired: 10 in]
                    n848 = To Quad Integer(1:w1358) -> (0:w1357:i64)
                    n849 = Unbundle(w1373) -> ("Real 2D Array[0]"=w1365:dbl, "Real 2D Array[1]"=w1364:dbl, "Real 2D Array[2]"=w1363:dbl, "Real 2D Array[3]"=w1362:dbl, "Real 2D Array[4]"=w1361:dbl)
                    n850 = Bundle(cluster=w1374, "hash"=w1370, "sys time"=w1357, "dt"=w1353, "x"=w1365, "y"=w1364, "speed"=w1363, "heading"=w1362, "yaw_rate"=w1361) -> (w1352:T12)
                    n851 = Flatten To String(anything=w1352, prepend array or string size? (T)=FALSE) -> (data string=w1368:string)  [unwired: 2 in, 2 out]
                    n852 = global read "rio_Global.vi" "LCM"() -> (w1367:T3)
                    n853 = call "LCM_send.vi"("DATA"=w1368, "ID"="POS_T", "LCM"=w1367) -> ()  [unwired: 7 in, 2 out]
                  }
                }
              }
            }
          }
        }
      }
      n854 = flat-sequence {
        frame #0 {
          n855 = while {
            shift-right: [w803] -> w798
            shift-left: refnum<visa-resource-name> "USB0::0x1546::0x01A8::NI-VISA-1003::1::RAW" ("VISA resource name") -> [w804]
            stop <- w802 continue-if-true
            n856 = VISA Open(VISA resource name=w804) -> (VISA resource name=w803:refnum<visa-resource-name>, error out=w802:errorcluster)  [unwired: 4 in]
          }
          n857 = VISA Clear(VISA resource name=w798) -> (VISA resource name out=w800:refnum<visa-resource-name>)  [unwired: 1 in, 1 out]
          n858 = property class="Instr"(reference=w800, "General Settings:Timeout Value"=u32 10) -> (reference out=→"gps1":refnum<visa-resource-name>)  [unwired: 1 in, 1 out]
        }
        frame #1 {
          n859 = while {
            stop <- FALSE stop-if-true
            n860 = local read "gps1"() -> (w807:refnum<visa-resource-name>)
            n861 = VISA Read(VISA resource name=w807, byte count=u32 100) -> (read buffer=w805:string)  [unwired: 1 in, 3 out]
            n862 = case shown="Default" w805 {
              selector: w805 -> [_ w810]
              frame "" {
                n863 = Wait (ms)(milliseconds to wait=u32 20) -> ()  [unwired: 1 out]
              }
              frame Default {
                n864 = local read "ecef ref"() -> (w811:dbl[])
                n865 = call "nmea.vi"("ecef ref"=w811, "NMEA"=w810) -> ("output"=w813:dbl[], "type"=w812:u32)  [unwired: 8 in]
                n866 = case shown="1" w812 {
                  tunnel: w813 -> [_ w815 w875]
                  frame 0, Default {
                  }
                  frame 1 {
                    n867 = global write "rio_Global.vi" "gps_pos 1"(w815) -> ()
                    n868 = Index Array(array=w815, index=1) -> (element=w817:dbl)
                    n869 = Not Equal To 0?(x=w817) -> (x != 0?=w814:bool)
                    n870 = case shown="True" w814 {
                      tunnel: w815 -> [_ w819]
                      frame False {
                      }
                      frame True {
                        n871 = First Call?() -> (First Call?: T/F=w818:bool)
                        n872 = case shown="True" w818 {
                          tunnel: w819 -> [w839 w852]
                          frame False {
                            n873 = Get Date/Time In Seconds() -> (seconds since 1Jan1904=w824:timestamp)
                            n874 = To Double Precision Float(number=w824) -> (double precision float=w823:dbl)
                            n875 = global read "rio_Global.vi" "LCM_GGA_T"() -> (w848:T14)
                            n876 = Array To Cluster(array=w839) -> (cluster=w847:T15)
                            n877 = Unbundle By Name(w848) -> ("hash"=w844:i64)
                            n878 = Multiply(x=w823, y=1000000.0) -> (x*y=w821:dbl)
                            n879 = Unbundle(w847) -> ("output[0]"=w849:dbl, "output[2]"=w838:dbl, "output[3]"=w837:dbl, "output[4]"=w836:dbl, "output[6]"=w835:dbl, "output[7]"=w833:dbl, "output[8]"=w831:dbl, "output[9]"=w829:dbl, "output[12]"=w828:dbl, "output[13]"=w827:dbl, "output[14]"=w826:dbl)  [unwired: 4 out]
                            n880 = local read "map name"() -> (w825:T1)
                            n881 = call "hash.vi"("input"=w844) -> ("output"=w843:i64)  [unwired: 10 in]
                            n882 = To Quad Integer(1:w821) -> (0:w820:i64)
                            n883 = To Long Integer(number=w835) -> (32bit integer=w834:i32)
                            n884 = To Long Integer(number=w833) -> (32bit integer=w832:i32)
                            n885 = To Long Integer(number=w831) -> (32bit integer=w830:i32)
                            n886 = Bundle(cluster=w848, "hash"=w843, "sys time"=w820, "time"=w849, "x"=w838, "y"=w837, "h"=w836, "numSV"=w834, "postype"=w832, "lag"=w830, "hordev"=w829, "lat"=w828, "lon"=w827, "hgt"=w826, "map_idx"=w825) -> (w845:T14)
                            n887 = Flatten To String(anything=w845, prepend array or string size? (T)=FALSE) -> (data string=w841:string)  [unwired: 2 in, 2 out]
                            n888 = global read "rio_Global.vi" "LCM"() -> (w840:T3)
                            n889 = call "LCM_send.vi"("DATA"=w841, "ID"="GGA_1", "LCM"=w840) -> ()  [unwired: 7 in, 2 out]
                          }
                          frame True {
                            n890 = Index Array(array=w852, index #1=12 ("index")) -> (element #1=w857:dbl, element #2=w861:dbl)  [unwired: 1 in]
                            n891 = for {
                              N: 11 -> [_]
                              tunnel: [w873] -> w863 mode=indexing
                              tunnel: [w872] -> w865 mode=indexing
                              i -> [w874]
                              n892 = call "getecefdcmref.vi"("map name"=w874) -> ("lat"=w873:dbl, "lon"=w872:dbl)  [unwired: 10 in, 3 out]
                            }
                            n893 = Multiply(x=w857, y=3.141592653589793) -> (x*y=w855:dbl)
                            n894 = Multiply(x=w861, y=3.141592653589793) -> (x*y=w859:dbl)
                            n895 = Divide(x=w855, y=180.0) -> (x/y=w864:dbl)
                            n896 = Divide(x=w859, y=180.0) -> (x/y=w866:dbl)
                            n897 = Subtract(x=w863, y=w864) -> (x-y=w867:dbl[])
                            n898 = Subtract(x=w865, y=w866) -> (x-y=w868:dbl[])
                            n899 = Square(x=w867) -> (x^2=w869:dbl[])
                            n900 = Square(x=w868) -> (x^2=w870:dbl[])
                            n901 = Add(x=w869, y=w870) -> (x+y=w871:dbl[])
                            n902 = Array Max & Min(array=w871) -> (min index (indices)=w850:i32)  [unwired: 3 out]
                            "map name" <- w850
                            n903 = call "getecefdcmref.vi"("map name"=w850) -> ("XYZ"=→"ecef ref":dbl[])  [unwired: 10 in, 4 out]
                          }
                        }
                      }
                    }
                  }
                  frame 2 {
                    n904 = flat-sequence {
                      tunnel: w875 -> [w877]
                      frame #0 {
                        n905 = Index Array(array=w877, index=1) -> (element=w879:dbl)
                        n906 = Not Equal To 0?(x=w879) -> (x != 0?=w876:bool)
                        n907 = case shown="True" w876 {
                          tunnel: w877 -> [_ w898]
                          frame False {
                          }
                          frame True {
                            n908 = Get Date/Time In Seconds() -> (seconds since 1Jan1904=w884:timestamp)
                            n909 = To Double Precision Float(number=w884) -> (double precision float=w883:dbl)
                            n910 = global read "rio_Global.vi" "LCM_RMC_T"() -> (w899:T16)
                            n911 = Unbundle By Name(w899) -> ("hash"=w895:i64)
                            n912 = Multiply(x=w883, y=1000000.0) -> (x*y=w881:dbl)
                            n913 = Array To Cluster(array=w898) -> (cluster=w897:T17)
                            n914 = To Quad Integer(1:w881) -> (0:w880:i64)
                            n915 = call "hash.vi"("input"=w895) -> ("output"=w894:i64)  [unwired: 10 in]
                            n916 = Unbundle(w897) -> ("output[0]"=w889:dbl, "output[2]"=w888:dbl, "output[4]"=w887:dbl, "output[5]"=w886:dbl, "output[6]"=w885:dbl)  [unwired: 2 out]
                            n917 = Bundle(cluster=w899, "hash"=w894, "sys time"=w880, "time"=w889, "speed"=w888, "heading"=w887, "lat"=w886, "lon"=w885) -> (w890:T16)
                            n918 = Flatten To String(anything=w890, prepend array or string size? (T)=FALSE) -> (data string=w892:string)  [unwired: 2 in, 2 out]
                            n919 = global read "rio_Global.vi" "LCM"() -> (w891:T3)
                            n920 = call "LCM_send.vi"("DATA"=w892, "ID"="RMC_1", "LCM"=w891) -> ()  [unwired: 7 in, 2 out]
                          }
                        }
                      }
                    }
                    n921 = global write "rio_Global.vi" "gps_vel 1"(w875) -> ()
                  }
                }
              }
            }
          }
        }
      }
    }
  }
